vi "Begin.vi"(8 "error in":errorcluster) -> (0 "error out":errorcluster)   [LabVIEW 2020]
doc: "Called before other user functions, this VI is expected to open initial I/O refnums, load in file data, and do all program initialization. Notice that the <B>error out</B> terminal is simply used for data flow. Wiring it to other structures or subVIs ensures that this VI runs first."
uses:
  <vilib>/Rock Robotics/WPI/ThirdParty/Phoenix-LabVIEW/Motor Controller/Controls/CTRE_Phoenix_MotorControl_SupplyCurrentLimitConfiguration.ctl
  <vilib>/Rock Robotics/WPI/DriverStation/WPI_DriverStationRobotMode2.ctl
  <vilib>/Rock Robotics/WPI/Joystick/WPI_JoystickDeviceEnum.ctl
  <vilib>/Rock Robotics/WPI/ThirdParty/REV Robotics/REVLib/Typedef/Spark MAX Status Frames.ctl
  <vilib>/Rock Robotics/WPI/ThirdParty/Phoenix-LabVIEW/Motor Controller/Controls/CTRE_Phoenix_MotorControl_StatusFrameEnhanced.ctl
  <vilib>/Rock Robotics/SystemInterfaces/DIO/FPGA_DIOPWMChannel.ctl
  <vilib>/Rock Robotics/WPI/ThirdParty/REV Robotics/REVLib/Typedef/Spark MAX Control Type.ctl
  <vilib>/Rock Robotics/WPI/ThirdParty/Phoenix-LabVIEW/Motor Controller/Controls/CTRE_Phoenix_MotorControl_TalonFXInvertType.ctl
  <vilib>/Rock Robotics/WPI/ThirdParty/REV Robotics/REVLib/Typedef/Spark MAX Sensor Type.ctl
  <vilib>/Rock Robotics/WPI/ThirdParty/REV Robotics/REVLib/Typedef/Spark MAX Motor Type.ctl
  <vilib>/Rock Robotics/WPI/ThirdParty/REV Robotics/REVLib/Typedef/Spark MAX Idle Mode.ctl
  <vilib>/Rock Robotics/WPI/ThirdParty/Phoenix-LabVIEW/Motor Controller/Controls/CTRE_Phoenix_MotorControl_ControlFrameEnhanced.ctl
  <vilib>/Rock Robotics/WPI/ThirdParty/Phoenix-LabVIEW/Pigeon IMU/CTRE_PigeonIMU_StatusFrameRate.ctl
  <vilib>/Rock Robotics/WPI/ThirdParty/Phoenix-LabVIEW/Motor Controller/Controls/CTRE_Phoenix_MotorControl_NeutralMode.ctl
  Robot Global Data.vi
  <vilib>/Rock Robotics/WPI/ThirdParty/Phoenix-LabVIEW/Pigeon IMU/CTRE_PigeonIMU_Open_CAN.vi
panel:
  in  "Supply Current Limit Configuration":T1={"Enable?"=TRUE, "Current Limit"=30.0, "Threshold Current"=0.0, "Threshold Time"=0.0}
  in  "configPath":path=path "/home/lvuser/Config/config.ini"
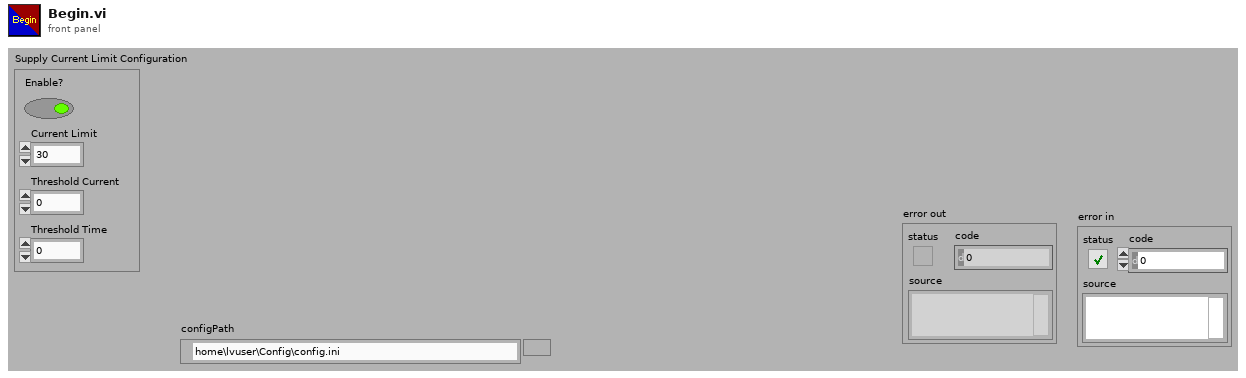
[diagram p1: front panel]
types:
  T1 = typedef "CTRE_Phoenix_MotorControl_SupplyCurrentLimitConfiguration.ctl" = cluster{"Enable?":bool, "Current Limit":dbl, "Threshold Current":dbl, "Threshold Time":dbl}
  T2 = typedef "WPI_DriverStationRobotMode2.ctl" = enum16{"Autonomous Disabled", "Autonomous Enabled", "Teleop Disabled", "Teleop Enabled", "Disconnected", "Finish", "Test Disabled", "Test Enabled", "Emergency Stopped"}
  T3 = typedef "CTRE_Phoenix_MotorControl_NeutralMode.ctl" = enum8{"EEPROMSetting", "Override to Coast", "Override to Brake"}
  T4 = typedef "Spark MAX Sensor Type.ctl" = enum16{"No Sensor", "Hall Sensor", "Encoder", "-Not Available-", "Analog", "Alternate Encoder"}
  T5 = typedef "CTRE_Phoenix_MotorControl_TalonFXInvertType.ctl" = enum16{"Counter-Clockwise", "Clockwise"}
  T6 = typedef "Spark MAX Status Frames.ctl" = enum16{"Status 0", "Status 1", "Status 2", "Status 3"}
  T7 = typedef "Spark MAX Idle Mode.ctl" = enum16{"Coast", "Brake"}
  T8 = typedef "Spark MAX Motor Type.ctl" = enum16{"Brushed", "Brushless"}
  T9 = cluster{"P Gain":dbl, "I Gain":dbl, "D Gain":dbl, "F Gain":dbl, "I Zone":dbl, "Min Output":dbl, "Max Output":dbl}
  T10 = typedef "Spark MAX Control Type.ctl" = enum16{"Percent VBus", "Voltage", "Velocity", "Position", "Smart Motion", "Current", "Smart Velocity"}
  T11 = typedef "FPGA_DIOPWMChannel.ctl" = enum8{"PWM 0", "PWM 1", "PWM 2", "PWM 3", "PWM 4", "PWM 5", "PWM 6", "PWM 7", "PWM 8", "PWM 9", "PWM MXP 0", "PWM MXP 1", "PWM MXP 2", "PWM MXP 3", "PWM MXP 4", "PWM MXP 5", "PWM MXP 6", "PWM MXP 7", "PWM MXP 8", "PWM MXP 9", "Invalid"}
  T12 = typedef "WPI_JoystickDeviceEnum.ctl" = enum16{"USB 0", "USB 1", "USB 2", "USB 3", "USB 4", "USB 5"}
  T13 = typedef "PiConfig.ctl" = cluster{"swerveModules":cluster{"leftFront":T14, "rightFront":T14, "leftRear":T14, "rightRear":T14}, "offsets":cluster{"leftFrontAngleOffset":dbl, "leftRearAngleOffset":dbl, "rightFrontAngleOffset":dbl, "rightRearAngleOffset":dbl}, "limits":cluster{"maxVelocity":dbl, "maxOverdriveVelocity":dbl, "maxAcceleration":dbl, "maxPickupVelocity":dbl, "maxClimbArmVelocity":dbl}, "speeds":cluster{"intakeSuckSpeed":dbl, "intakeSpitSpeed":dbl, "indexerSuckSpeed":dbl, "indexerSpitSpeed":dbl, "indexerShootSpeed":dbl, "indexerBumpBackSpeed":dbl, "shooterSpinupSpeed":dbl, "kickupSpinupSpeed":dbl, "shooterLowShootSpeed":dbl, "shooterHighShootSpeed":dbl, "shooterPadSpeed":dbl, "shooterWallSpeed":dbl}, "positions":cluster{"intakeStarting":dbl, "intakeStow":dbl, "intakeSuck":dbl, "armPounce":dbl, "armStow":dbl, "armUp":dbl, "winchPounce":dbl, "winchOut":dbl, "winchStow":dbl, "intakeSpit":dbl, "winchBarEngage":dbl, "winchBottomClimb":dbl, "hoodHighShoot":dbl, "armClearHooks":dbl, "winchClearHooks":dbl, "armLiftNextBar":dbl, "winchEngageHooksNextBar":dbl, "winchEngagePassive":dbl, "winchTraversalClimb":dbl, "hoodPadShoot":dbl, "turretPadShoot":dbl, "hoodWallShoot":dbl, "turretWallShoot":dbl, "winchRobotOffBar":dbl, "winchSettleClimb":dbl}, "inversions":cluster{"rightShooter":bool, "leftShooter":bool}}
  T14 = typedef "Swerve Module Parameters.ctl" = cluster{"driveCANID":dbl, "angleCANID":i32, "canCoderCANID":dbl, "moduleName":string, "driveMotorNeutralMode":T3, "driveCurrentLimitConfig":T1, "driveFeedbackDevice":T15, "driveInitialSensorPosition":dbl, "driveEnableVoltageComp":bool, "driveVoltageComp":dbl, "driveRampRate":dbl, "angleCurrentLimit":dbl, "angleSensorType":T4, "angleMotorType":T8, "angleConversionFactor":dbl, "anglePIDRamp":dbl, "angleVoltageComp":dbl, "angleIdleMode":T7, "cancoderConfig":T16, "angleInitialSensorPosition":dbl}
  T15 = typedef "CTRE_Phoenix_MotorControl_FeedbackDevice_TalonFX.ctl" = i8
  T16 = typedef "CTRE_Phoenix_CANcoder_Configurables.ctl" = cluster{"Sensor Initialization Strategy":T17, "Absolute Sensor Range":T18, "Velocity Measurement Period":T19, "Velocity Measurement Window":i32, "Magnet Offset (Degrees)":dbl, "Sensor Direction":bool, "Sensor Coefficient":dbl, "Unit String":string, "Sensor Time Base":T20}
  T17 = typedef "CTRE_Phoenix_CANcoder_SensorInitializationStrategy.ctl" = enum16{"Boot To Zero", "Boot To Absolute Position"}
  T18 = typedef "CTRE_Phoenix_CANcoder_AbsoluteSensorRange.ctl" = enum16{"Unsigned [0 to 360)", "Signed [-180 to +180)"}
  T19 = typedef "CTRE_Phoenix_MotorControl_VelocityMeasurementPeriod.ctl" = u16
  T20 = typedef "CTRE_Phoenix_CANcoder_SensorTimeBase.ctl" = enum16{"Per100Ms_Legacy", "PerSecond", "PerMinute"}
  T21 = typedef "CTRE_Phoenix_MotorControl_ControlFrameEnhanced.ctl" = u32
  T22 = typedef "CTRE_Phoenix_MotorControl_StatusFrameEnhanced.ctl" = u16
  T23 = typedef "CTRE_PigeonIMU_StatusFrameRate.ctl" = u32
  T24 = typedef "WPI_JoystickDevRef.ctl" = cluster{"Device":T12}
  T25 = typedef "WPI_ServoDeviceRef.ctl" = cluster{"DeviceStatus":errorcluster, "PWM Channel":T11, "DeadBand":T26}
  T26 = typedef "WPI_PWMDeadband.ctl" = cluster{"Name":string, "maxPositivePwm":i32, "minPositivePwm":i32, "centerPwm":i32, "maxNegativePwm":i32, "minNegativePwm":i32, "angularRange":u16}
  T27 = typedef "CTRE_PigeonIMU_DeviceRef.ctl" = cluster{"DeviceStatus":errorcluster, "Device Number":u8, "Type":T28, "Device ID":u32, "Handle":u64, "UsageFrame":u32, "Library Path":path}
  T28 = typedef "CTRE_PigeonIMU_ConnectionType.ctl" = u32
  T29 = typedef "WPI_MotorControlDeviceRef.ctl" = cluster{"DeviceStatus":errorcluster, "Type":T30, "PWM":cluster{"PWM Channel":T11, "DeadBand":T26}, "CAN":cluster{"Device Number":u8, "SetOutput VI Ref":variant, "GetOutput VI Ref":variant, "Enable VI Ref":variant, "Disable VI Ref":variant, "Data":variant}, "Invert":bool, "DIO PWM":cluster{"PWM \"Enable\" Channel":T11, "DIOChannel":T31, "PWM Rate":dbl}}
  T30 = typedef "WPI_MotorControlType.ctl" = enum16{"PWM", "CAN", "DIO PWM"}
  T31 = typedef "FPGA_DIOChannel.ctl" = enum8{"DIO 0", "DIO 1", "DIO 2", "DIO 3", "DIO 4", "DIO 5", "DIO 6", "DIO 7", "DIO 8", "DIO 9", "DIO MXP 0", "DIO MXP 1", "DIO MXP 2", "DIO MXP 3", "DIO MXP 4", "DIO MXP 5", "DIO MXP 6", "DIO MXP 7", "DIO MXP 8", "DIO MXP 9", "DIO MXP 10", "DIO MXP 11", "DIO MXP 12", "DIO MXP 13", "DIO MXP 14", "DIO MXP 15", "SPI Port CS1", "SPI Port CS2", "SPI Port CS3", "SPI Port MISO", "SPI Port MOSI", "Invalid"}
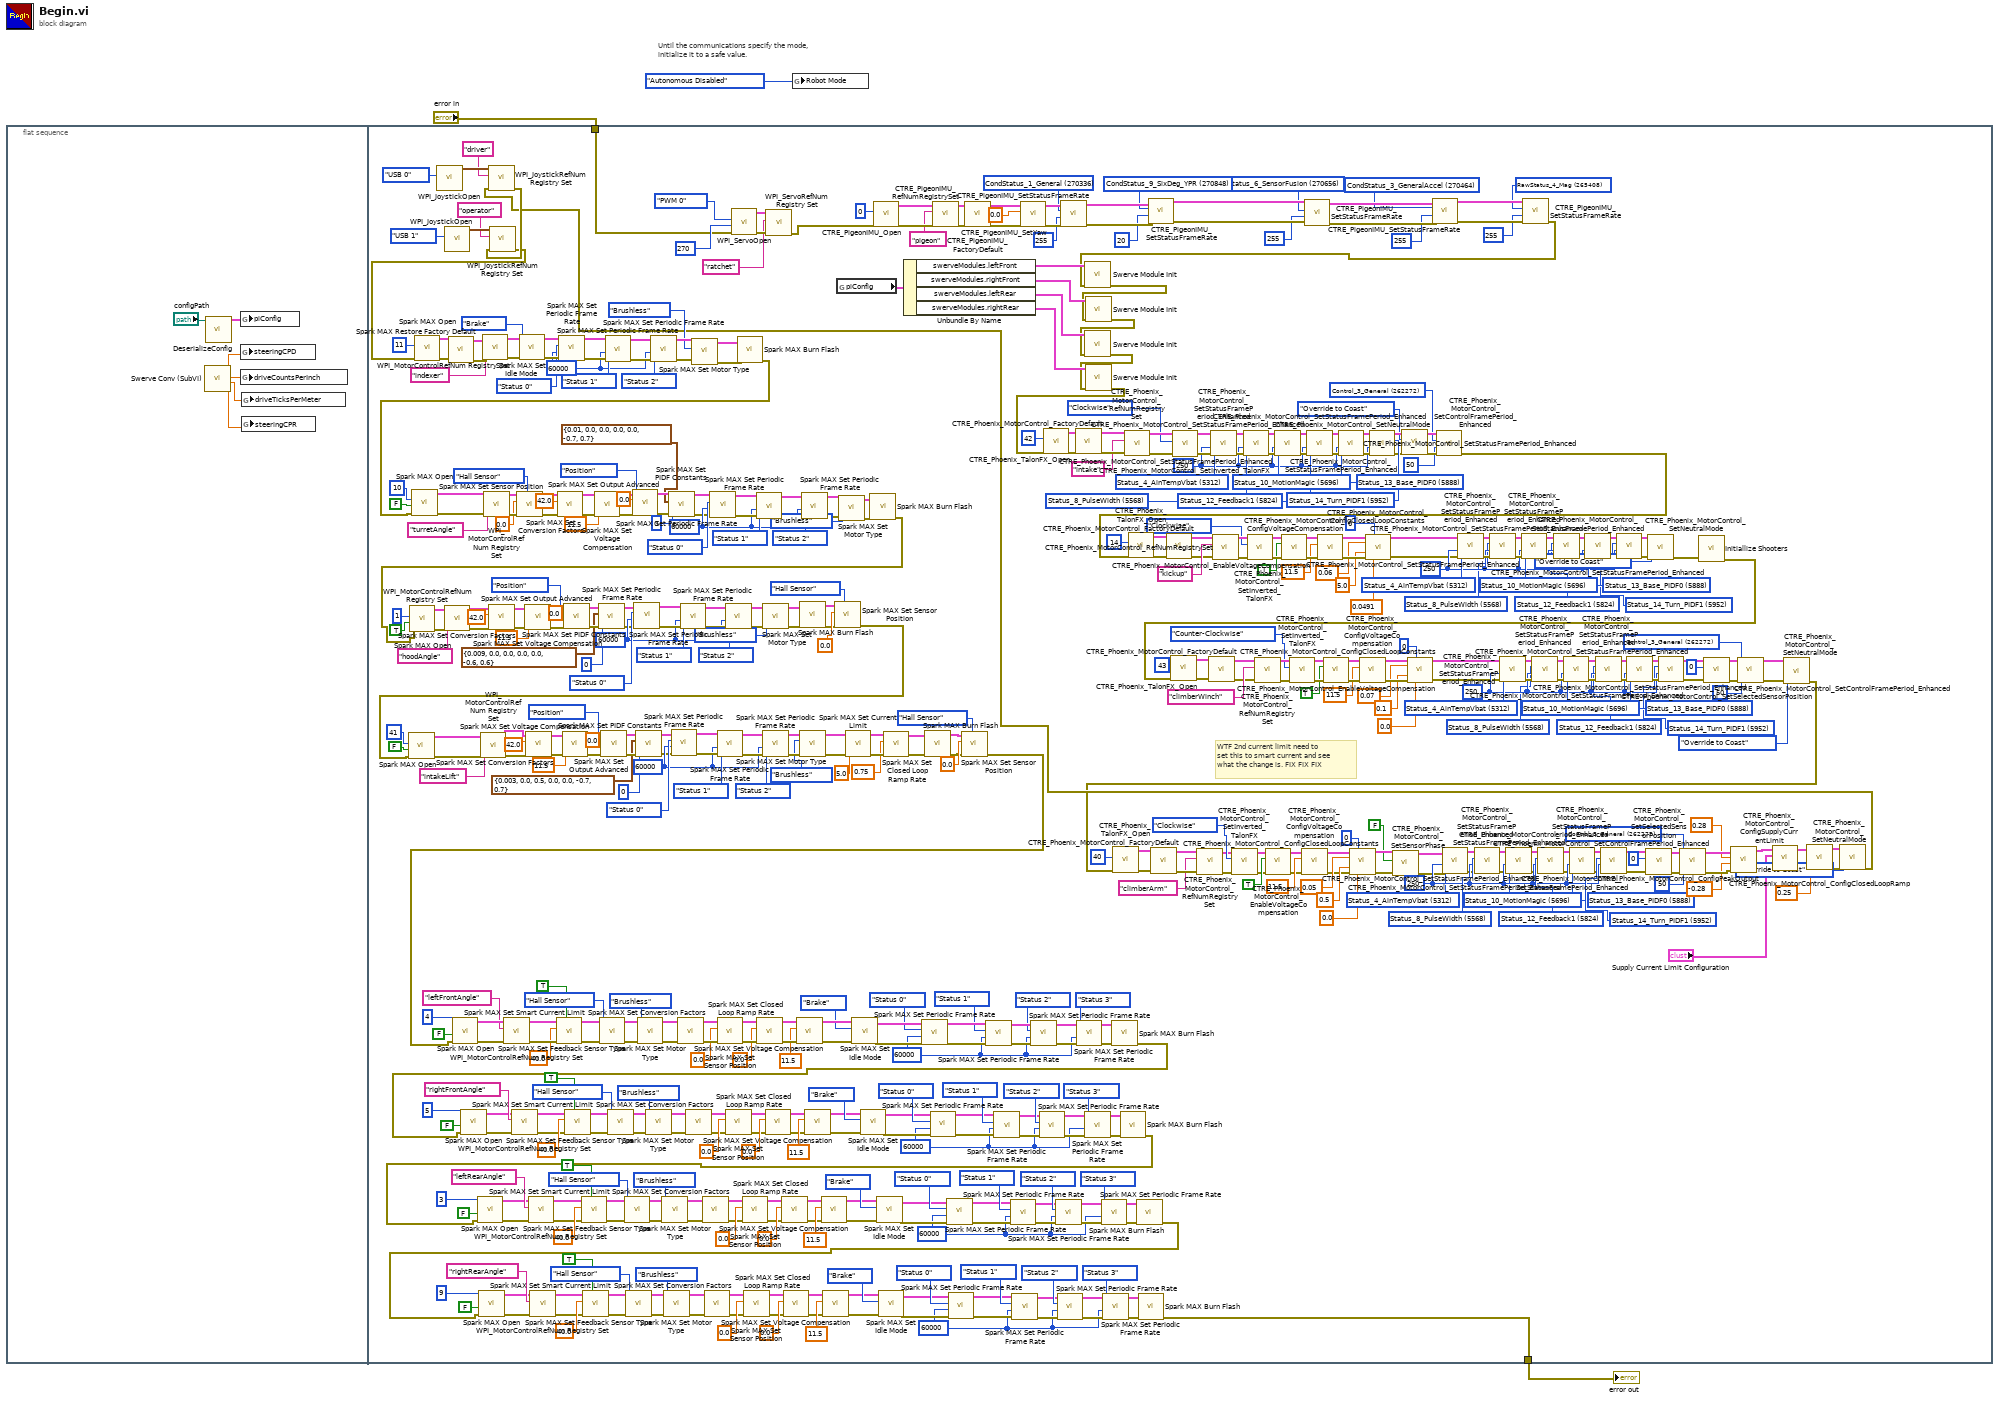
[diagram p0: block diagram]
diagram:
  # "Until the communications specify the mode,\ninitialize it to a safe value."
  n1 = flat-sequence {
    tunnel: "error in" -> [w97]
    tunnel: [w91] -> w1
    frame #0 {
      n2 = call "Swerve Conv (SubVI).vi"() -> ("steeringModuleCPR"=w8:dbl, "driveCountsPerMeter"=w4:dbl, "driveCountsPerInch"=w6:dbl, "steeringModuleCPD"=w7:dbl)  [unwired: 8 in]
      n3 = call "DeserializeConfig.vi"("configPath"="configPath") -> ("config"=w9:T13)  [unwired: 10 in]
      n4 = global write "Robot Global Data.vi" "piConfig"(w9) -> ()
      n5 = global write "Robot Global Data.vi" "steeringCPD"(w7) -> ()
      n6 = global write "Robot Global Data.vi" "driveCountsPerInch"(w6) -> ()
      n7 = global write "Robot Global Data.vi" "driveTicksPerMeter"(w4) -> ()
      n8 = global write "Robot Global Data.vi" "steeringCPR"(w8) -> ()
    }
    frame #1 {
      w89 = T21 262272 items=["Control_3_General"=262272, "Control_4_Advanced"=262336, "Control_5_FeedbackOutputOverride"=262400, "Control_6_MotProfAddTrajPoint"=262464] ("Control Frame")
      w77 = 250 ("periodMs")
      w80 = T22 5952 items=["Status_1_General"=5120, "Status_2_Feedback0"=5184, "Status_3_Quadrature"=5248, "Status_4_AinTempVbat"=5312, "Status_6_Misc"=5440, "Status_7_CommStatus"=5504, "Status_8_PulseWidth"=5568, "Status_9_MotProfBuffer"=5632, "Status_10_MotionMagic"=5696, "Status_11_UartGadgeteer"=5760, "Status_12_Feedback1"=5824, "Status_13_Base_PIDF0"=5888, "Status_14_Turn_PIDF1"=5952, "Status_15_FirmwareApiStatus"=6016, "Status_Brushless_Current"=4672] ("Status Frame")
      w76 = T22 5888 items=["Status_1_General"=5120, "Status_2_Feedback0"=5184, "Status_3_Quadrature"=5248, "Status_4_AinTempVbat"=5312, "Status_6_Misc"=5440, "Status_7_CommStatus"=5504, "Status_8_PulseWidth"=5568, "Status_9_MotProfBuffer"=5632, "Status_10_MotionMagic"=5696, "Status_11_UartGadgeteer"=5760, "Status_12_Feedback1"=5824, "Status_13_Base_PIDF0"=5888, "Status_14_Turn_PIDF1"=5952, "Status_15_FirmwareApiStatus"=6016, "Status_Brushless_Current"=4672] ("Status Frame")
      w79 = T22 5824 items=["Status_1_General"=5120, "Status_2_Feedback0"=5184, "Status_3_Quadrature"=5248, "Status_4_AinTempVbat"=5312, "Status_6_Misc"=5440, "Status_7_CommStatus"=5504, "Status_8_PulseWidth"=5568, "Status_9_MotProfBuffer"=5632, "Status_10_MotionMagic"=5696, "Status_11_UartGadgeteer"=5760, "Status_12_Feedback1"=5824, "Status_13_Base_PIDF0"=5888, "Status_14_Turn_PIDF1"=5952, "Status_15_FirmwareApiStatus"=6016, "Status_Brushless_Current"=4672] ("Status Frame")
      w75 = T22 5696 items=["Status_1_General"=5120, "Status_2_Feedback0"=5184, "Status_3_Quadrature"=5248, "Status_4_AinTempVbat"=5312, "Status_6_Misc"=5440, "Status_7_CommStatus"=5504, "Status_8_PulseWidth"=5568, "Status_9_MotProfBuffer"=5632, "Status_10_MotionMagic"=5696, "Status_11_UartGadgeteer"=5760, "Status_12_Feedback1"=5824, "Status_13_Base_PIDF0"=5888, "Status_14_Turn_PIDF1"=5952, "Status_15_FirmwareApiStatus"=6016, "Status_Brushless_Current"=4672] ("Status Frame")
      w78 = T22 5568 items=["Status_1_General"=5120, "Status_2_Feedback0"=5184, "Status_3_Quadrature"=5248, "Status_4_AinTempVbat"=5312, "Status_6_Misc"=5440, "Status_7_CommStatus"=5504, "Status_8_PulseWidth"=5568, "Status_9_MotProfBuffer"=5632, "Status_10_MotionMagic"=5696, "Status_11_UartGadgeteer"=5760, "Status_12_Feedback1"=5824, "Status_13_Base_PIDF0"=5888, "Status_14_Turn_PIDF1"=5952, "Status_15_FirmwareApiStatus"=6016, "Status_Brushless_Current"=4672] ("Status Frame")
      w74 = T22 5312 items=["Status_1_General"=5120, "Status_2_Feedback0"=5184, "Status_3_Quadrature"=5248, "Status_4_AinTempVbat"=5312, "Status_6_Misc"=5440, "Status_7_CommStatus"=5504, "Status_8_PulseWidth"=5568, "Status_9_MotProfBuffer"=5632, "Status_10_MotionMagic"=5696, "Status_11_UartGadgeteer"=5760, "Status_12_Feedback1"=5824, "Status_13_Base_PIDF0"=5888, "Status_14_Turn_PIDF1"=5952, "Status_15_FirmwareApiStatus"=6016, "Status_Brushless_Current"=4672] ("Status Frame")
      w102 = T23 265408 items=["CondStatus_1_General"=270336, "CondStatus_9_SixDeg_YPR"=270848, "CondStatus_6_SensorFusion"=270656, "CondStatus_11_GyroAccum"=270976, "CondStatus_2_GeneralCompass"=270400, "CondStatus_3_GeneralAccel"=270464, "CondStatus_10_SixDeg_Quat"=270912, "RawStatus_4_Mag"=265408, "BiasedStatus_2_Gyro"=269376, "BiasedStatus_4_Mag"=269504, "BiasedStatus_6_Accel"=269632] ("StatusFrame")
      w103 = T23 270464 items=["CondStatus_1_General"=270336, "CondStatus_9_SixDeg_YPR"=270848, "CondStatus_6_SensorFusion"=270656, "CondStatus_11_GyroAccum"=270976, "CondStatus_2_GeneralCompass"=270400, "CondStatus_3_GeneralAccel"=270464, "CondStatus_10_SixDeg_Quat"=270912, "RawStatus_4_Mag"=265408, "BiasedStatus_2_Gyro"=269376, "BiasedStatus_4_Mag"=269504, "BiasedStatus_6_Accel"=269632] ("StatusFrame")
      w104 = T23 270656 items=["CondStatus_1_General"=270336, "CondStatus_9_SixDeg_YPR"=270848, "CondStatus_6_SensorFusion"=270656, "CondStatus_11_GyroAccum"=270976, "CondStatus_2_GeneralCompass"=270400, "CondStatus_3_GeneralAccel"=270464, "CondStatus_10_SixDeg_Quat"=270912, "RawStatus_4_Mag"=265408, "BiasedStatus_2_Gyro"=269376, "BiasedStatus_4_Mag"=269504, "BiasedStatus_6_Accel"=269632] ("StatusFrame")
      w105 = T23 270848 items=["CondStatus_1_General"=270336, "CondStatus_9_SixDeg_YPR"=270848, "CondStatus_6_SensorFusion"=270656, "CondStatus_11_GyroAccum"=270976, "CondStatus_2_GeneralCompass"=270400, "CondStatus_3_GeneralAccel"=270464, "CondStatus_10_SixDeg_Quat"=270912, "RawStatus_4_Mag"=265408, "BiasedStatus_2_Gyro"=269376, "BiasedStatus_4_Mag"=269504, "BiasedStatus_6_Accel"=269632] ("StatusFrame")
      w115 = T23 270336 items=["CondStatus_1_General"=270336, "CondStatus_9_SixDeg_YPR"=270848, "CondStatus_6_SensorFusion"=270656, "CondStatus_11_GyroAccum"=270976, "CondStatus_2_GeneralCompass"=270400, "CondStatus_3_GeneralAccel"=270464, "CondStatus_10_SixDeg_Quat"=270912, "RawStatus_4_Mag"=265408, "BiasedStatus_2_Gyro"=269376, "BiasedStatus_4_Mag"=269504, "BiasedStatus_6_Accel"=269632] ("StatusFrame")
      w119 = T21 262272 items=["Control_3_General"=262272, "Control_4_Advanced"=262336, "Control_5_FeedbackOutputOverride"=262400, "Control_6_MotProfAddTrajPoint"=262464] ("Control Frame")
      w123 = T21 262272 items=["Control_3_General"=262272, "Control_4_Advanced"=262336, "Control_5_FeedbackOutputOverride"=262400, "Control_6_MotProfAddTrajPoint"=262464] ("Control Frame")
      w131 = u16 60000 ("Frame rate (ms)")
      w132 = u16 60000 ("Frame rate (ms)")
      w133 = u16 60000 ("Frame rate (ms)")
      w134 = u16 60000 ("Frame rate (ms)")
      w332 = 250 ("periodMs")
      w329 = T22 5952 items=["Status_1_General"=5120, "Status_2_Feedback0"=5184, "Status_3_Quadrature"=5248, "Status_4_AinTempVbat"=5312, "Status_6_Misc"=5440, "Status_7_CommStatus"=5504, "Status_8_PulseWidth"=5568, "Status_9_MotProfBuffer"=5632, "Status_10_MotionMagic"=5696, "Status_11_UartGadgeteer"=5760, "Status_12_Feedback1"=5824, "Status_13_Base_PIDF0"=5888, "Status_14_Turn_PIDF1"=5952, "Status_15_FirmwareApiStatus"=6016, "Status_Brushless_Current"=4672] ("Status Frame")
      w333 = T22 5888 items=["Status_1_General"=5120, "Status_2_Feedback0"=5184, "Status_3_Quadrature"=5248, "Status_4_AinTempVbat"=5312, "Status_6_Misc"=5440, "Status_7_CommStatus"=5504, "Status_8_PulseWidth"=5568, "Status_9_MotProfBuffer"=5632, "Status_10_MotionMagic"=5696, "Status_11_UartGadgeteer"=5760, "Status_12_Feedback1"=5824, "Status_13_Base_PIDF0"=5888, "Status_14_Turn_PIDF1"=5952, "Status_15_FirmwareApiStatus"=6016, "Status_Brushless_Current"=4672] ("Status Frame")
      w330 = T22 5824 items=["Status_1_General"=5120, "Status_2_Feedback0"=5184, "Status_3_Quadrature"=5248, "Status_4_AinTempVbat"=5312, "Status_6_Misc"=5440, "Status_7_CommStatus"=5504, "Status_8_PulseWidth"=5568, "Status_9_MotProfBuffer"=5632, "Status_10_MotionMagic"=5696, "Status_11_UartGadgeteer"=5760, "Status_12_Feedback1"=5824, "Status_13_Base_PIDF0"=5888, "Status_14_Turn_PIDF1"=5952, "Status_15_FirmwareApiStatus"=6016, "Status_Brushless_Current"=4672] ("Status Frame")
      w334 = T22 5696 items=["Status_1_General"=5120, "Status_2_Feedback0"=5184, "Status_3_Quadrature"=5248, "Status_4_AinTempVbat"=5312, "Status_6_Misc"=5440, "Status_7_CommStatus"=5504, "Status_8_PulseWidth"=5568, "Status_9_MotProfBuffer"=5632, "Status_10_MotionMagic"=5696, "Status_11_UartGadgeteer"=5760, "Status_12_Feedback1"=5824, "Status_13_Base_PIDF0"=5888, "Status_14_Turn_PIDF1"=5952, "Status_15_FirmwareApiStatus"=6016, "Status_Brushless_Current"=4672] ("Status Frame")
      w331 = T22 5568 items=["Status_1_General"=5120, "Status_2_Feedback0"=5184, "Status_3_Quadrature"=5248, "Status_4_AinTempVbat"=5312, "Status_6_Misc"=5440, "Status_7_CommStatus"=5504, "Status_8_PulseWidth"=5568, "Status_9_MotProfBuffer"=5632, "Status_10_MotionMagic"=5696, "Status_11_UartGadgeteer"=5760, "Status_12_Feedback1"=5824, "Status_13_Base_PIDF0"=5888, "Status_14_Turn_PIDF1"=5952, "Status_15_FirmwareApiStatus"=6016, "Status_Brushless_Current"=4672] ("Status Frame")
      w335 = T22 5312 items=["Status_1_General"=5120, "Status_2_Feedback0"=5184, "Status_3_Quadrature"=5248, "Status_4_AinTempVbat"=5312, "Status_6_Misc"=5440, "Status_7_CommStatus"=5504, "Status_8_PulseWidth"=5568, "Status_9_MotProfBuffer"=5632, "Status_10_MotionMagic"=5696, "Status_11_UartGadgeteer"=5760, "Status_12_Feedback1"=5824, "Status_13_Base_PIDF0"=5888, "Status_14_Turn_PIDF1"=5952, "Status_15_FirmwareApiStatus"=6016, "Status_Brushless_Current"=4672] ("Status Frame")
      w370 = u16 60000 ("Frame rate (ms)")
      w421 = 250 ("periodMs")
      w418 = T22 5952 items=["Status_1_General"=5120, "Status_2_Feedback0"=5184, "Status_3_Quadrature"=5248, "Status_4_AinTempVbat"=5312, "Status_6_Misc"=5440, "Status_7_CommStatus"=5504, "Status_8_PulseWidth"=5568, "Status_9_MotProfBuffer"=5632, "Status_10_MotionMagic"=5696, "Status_11_UartGadgeteer"=5760, "Status_12_Feedback1"=5824, "Status_13_Base_PIDF0"=5888, "Status_14_Turn_PIDF1"=5952, "Status_15_FirmwareApiStatus"=6016, "Status_Brushless_Current"=4672] ("Status Frame")
      w422 = T22 5888 items=["Status_1_General"=5120, "Status_2_Feedback0"=5184, "Status_3_Quadrature"=5248, "Status_4_AinTempVbat"=5312, "Status_6_Misc"=5440, "Status_7_CommStatus"=5504, "Status_8_PulseWidth"=5568, "Status_9_MotProfBuffer"=5632, "Status_10_MotionMagic"=5696, "Status_11_UartGadgeteer"=5760, "Status_12_Feedback1"=5824, "Status_13_Base_PIDF0"=5888, "Status_14_Turn_PIDF1"=5952, "Status_15_FirmwareApiStatus"=6016, "Status_Brushless_Current"=4672] ("Status Frame")
      w419 = T22 5824 items=["Status_1_General"=5120, "Status_2_Feedback0"=5184, "Status_3_Quadrature"=5248, "Status_4_AinTempVbat"=5312, "Status_6_Misc"=5440, "Status_7_CommStatus"=5504, "Status_8_PulseWidth"=5568, "Status_9_MotProfBuffer"=5632, "Status_10_MotionMagic"=5696, "Status_11_UartGadgeteer"=5760, "Status_12_Feedback1"=5824, "Status_13_Base_PIDF0"=5888, "Status_14_Turn_PIDF1"=5952, "Status_15_FirmwareApiStatus"=6016, "Status_Brushless_Current"=4672] ("Status Frame")
      w423 = T22 5696 items=["Status_1_General"=5120, "Status_2_Feedback0"=5184, "Status_3_Quadrature"=5248, "Status_4_AinTempVbat"=5312, "Status_6_Misc"=5440, "Status_7_CommStatus"=5504, "Status_8_PulseWidth"=5568, "Status_9_MotProfBuffer"=5632, "Status_10_MotionMagic"=5696, "Status_11_UartGadgeteer"=5760, "Status_12_Feedback1"=5824, "Status_13_Base_PIDF0"=5888, "Status_14_Turn_PIDF1"=5952, "Status_15_FirmwareApiStatus"=6016, "Status_Brushless_Current"=4672] ("Status Frame")
      w420 = T22 5568 items=["Status_1_General"=5120, "Status_2_Feedback0"=5184, "Status_3_Quadrature"=5248, "Status_4_AinTempVbat"=5312, "Status_6_Misc"=5440, "Status_7_CommStatus"=5504, "Status_8_PulseWidth"=5568, "Status_9_MotProfBuffer"=5632, "Status_10_MotionMagic"=5696, "Status_11_UartGadgeteer"=5760, "Status_12_Feedback1"=5824, "Status_13_Base_PIDF0"=5888, "Status_14_Turn_PIDF1"=5952, "Status_15_FirmwareApiStatus"=6016, "Status_Brushless_Current"=4672] ("Status Frame")
      w424 = T22 5312 items=["Status_1_General"=5120, "Status_2_Feedback0"=5184, "Status_3_Quadrature"=5248, "Status_4_AinTempVbat"=5312, "Status_6_Misc"=5440, "Status_7_CommStatus"=5504, "Status_8_PulseWidth"=5568, "Status_9_MotProfBuffer"=5632, "Status_10_MotionMagic"=5696, "Status_11_UartGadgeteer"=5760, "Status_12_Feedback1"=5824, "Status_13_Base_PIDF0"=5888, "Status_14_Turn_PIDF1"=5952, "Status_15_FirmwareApiStatus"=6016, "Status_Brushless_Current"=4672] ("Status Frame")
      w435 = 250 ("periodMs")
      w436 = T22 5952 items=["Status_1_General"=5120, "Status_2_Feedback0"=5184, "Status_3_Quadrature"=5248, "Status_4_AinTempVbat"=5312, "Status_6_Misc"=5440, "Status_7_CommStatus"=5504, "Status_8_PulseWidth"=5568, "Status_9_MotProfBuffer"=5632, "Status_10_MotionMagic"=5696, "Status_11_UartGadgeteer"=5760, "Status_12_Feedback1"=5824, "Status_13_Base_PIDF0"=5888, "Status_14_Turn_PIDF1"=5952, "Status_15_FirmwareApiStatus"=6016, "Status_Brushless_Current"=4672] ("Status Frame")
      w437 = T22 5888 items=["Status_1_General"=5120, "Status_2_Feedback0"=5184, "Status_3_Quadrature"=5248, "Status_4_AinTempVbat"=5312, "Status_6_Misc"=5440, "Status_7_CommStatus"=5504, "Status_8_PulseWidth"=5568, "Status_9_MotProfBuffer"=5632, "Status_10_MotionMagic"=5696, "Status_11_UartGadgeteer"=5760, "Status_12_Feedback1"=5824, "Status_13_Base_PIDF0"=5888, "Status_14_Turn_PIDF1"=5952, "Status_15_FirmwareApiStatus"=6016, "Status_Brushless_Current"=4672] ("Status Frame")
      w438 = T22 5824 items=["Status_1_General"=5120, "Status_2_Feedback0"=5184, "Status_3_Quadrature"=5248, "Status_4_AinTempVbat"=5312, "Status_6_Misc"=5440, "Status_7_CommStatus"=5504, "Status_8_PulseWidth"=5568, "Status_9_MotProfBuffer"=5632, "Status_10_MotionMagic"=5696, "Status_11_UartGadgeteer"=5760, "Status_12_Feedback1"=5824, "Status_13_Base_PIDF0"=5888, "Status_14_Turn_PIDF1"=5952, "Status_15_FirmwareApiStatus"=6016, "Status_Brushless_Current"=4672] ("Status Frame")
      w439 = T22 5696 items=["Status_1_General"=5120, "Status_2_Feedback0"=5184, "Status_3_Quadrature"=5248, "Status_4_AinTempVbat"=5312, "Status_6_Misc"=5440, "Status_7_CommStatus"=5504, "Status_8_PulseWidth"=5568, "Status_9_MotProfBuffer"=5632, "Status_10_MotionMagic"=5696, "Status_11_UartGadgeteer"=5760, "Status_12_Feedback1"=5824, "Status_13_Base_PIDF0"=5888, "Status_14_Turn_PIDF1"=5952, "Status_15_FirmwareApiStatus"=6016, "Status_Brushless_Current"=4672] ("Status Frame")
      w440 = T22 5568 items=["Status_1_General"=5120, "Status_2_Feedback0"=5184, "Status_3_Quadrature"=5248, "Status_4_AinTempVbat"=5312, "Status_6_Misc"=5440, "Status_7_CommStatus"=5504, "Status_8_PulseWidth"=5568, "Status_9_MotProfBuffer"=5632, "Status_10_MotionMagic"=5696, "Status_11_UartGadgeteer"=5760, "Status_12_Feedback1"=5824, "Status_13_Base_PIDF0"=5888, "Status_14_Turn_PIDF1"=5952, "Status_15_FirmwareApiStatus"=6016, "Status_Brushless_Current"=4672] ("Status Frame")
      w441 = T22 5312 items=["Status_1_General"=5120, "Status_2_Feedback0"=5184, "Status_3_Quadrature"=5248, "Status_4_AinTempVbat"=5312, "Status_6_Misc"=5440, "Status_7_CommStatus"=5504, "Status_8_PulseWidth"=5568, "Status_9_MotProfBuffer"=5632, "Status_10_MotionMagic"=5696, "Status_11_UartGadgeteer"=5760, "Status_12_Feedback1"=5824, "Status_13_Base_PIDF0"=5888, "Status_14_Turn_PIDF1"=5952, "Status_15_FirmwareApiStatus"=6016, "Status_Brushless_Current"=4672] ("Status Frame")
      w458 = u16 60000 ("Frame rate (ms)")
      w466 = u16 60000 ("Frame rate (ms)")
      w474 = u16 60000 ("Frame rate (ms)")
      # "WTF 2nd current limit need to\nset this to smart current and see\nwhat the change is. FIX FIX FIX"
      n9 = call <vilib>:"WPI_JoystickOpen.vi"("JoystickDevice"=WPI_JoystickDeviceEnum."USB 0") -> ("JoystickDevRef"=w578:T24)  [unwired: 10 in]
      n10 = call <vilib>:"WPI_JoystickOpen.vi"("JoystickDevice"=WPI_JoystickDeviceEnum."USB 1") -> ("JoystickDevRef"=w579:T24)  [unwired: 10 in]
      n11 = call <vilib>:"WPI_ServoOpen.vi"("error in (no error)"=w97, "Angular Range"=u16 270, "PWM Channel"=FPGA_DIOPWMChannel."PWM 0") -> ("error out"=w397:errorcluster, "ServoDeviceRef"=w396:T25)  [unwired: 7 in]
      n12 = call <vilib>:"WPI_ServoRefNum Registry Set.vi"("error in (no error)"=w397, "refnum name"="ratchet", "ServoDeviceRef"=w396) -> ("error out"=w96:errorcluster)  [unwired: 7 in, 1 out]
      n13 = global read "Robot Global Data.vi" "piConfig"() -> (w573:T13)
      n14 = call-poly <vilib>:"CTRE_PigeonIMU_Open.vi"("error in"=w96, "Device Number"=u8 0) -> ("error out"=w582:errorcluster, "PigeonIMUDevRef"=w583:T27)  [unwired: 8 in]
      n15 = Unbundle By Name(w573) -> ("swerveModules.leftFront"=w572:T14, "swerveModules.rightFront"=w571:T14, "swerveModules.leftRear"=w569:T14, "swerveModules.rightRear"=w570:T14)
      n16 = call <vilib>:"CTRE_PigeonIMU_RefNumRegistrySet.vi"("error in (no error)"=w582, "refnum name"="pigeon", "PigeonIMUDevRef"=w583) -> ("error out"=w584:errorcluster, "PigeonIMUDevRef"=w585:T27)  [unwired: 7 in]
      n17 = call <vilib>:"CTRE_PigeonIMU_FactoryDefault.vi"("error in"=w584, "PigeonIMUDevRef"=w585) -> ("error out"=w586:errorcluster, "PigeonIMUDevRef"=w587:T27)  [unwired: 8 in]
      n18 = call <vilib>:"CTRE_PigeonIMU_SetYaw.vi"("error in (no error)"=w586, "Value"=0.0, "PigeonIMUDevRef"=w587) -> ("error out"=w117:errorcluster, "PigeonIMUDevRef"=w116:T27)  [unwired: 7 in]
      n19 = call <vilib>:"CTRE_PigeonIMU_SetStatusFrameRate.vi"("error in (no error)"=w117, "Period (ms)"=i16 255, "StatusFrame"=w115, "PigeonIMUDevRef"=w116) -> ("error out"=w111:errorcluster, "PigeonIMUDevRef"=w112:T27)  [unwired: 6 in]
      n20 = call <vilib>:"CTRE_PigeonIMU_SetStatusFrameRate.vi"("error in (no error)"=w111, "Period (ms)"=i16 20, "StatusFrame"=w105, "PigeonIMUDevRef"=w112) -> ("error out"=w109:errorcluster, "PigeonIMUDevRef"=w110:T27)  [unwired: 6 in]
      n21 = call <vilib>:"CTRE_PigeonIMU_SetStatusFrameRate.vi"("error in (no error)"=w109, "Period (ms)"=i16 255, "StatusFrame"=w104, "PigeonIMUDevRef"=w110) -> ("error out"=w114:errorcluster, "PigeonIMUDevRef"=w113:T27)  [unwired: 6 in]
      n22 = call <vilib>:"CTRE_PigeonIMU_SetStatusFrameRate.vi"("error in (no error)"=w114, "Period (ms)"=i16 255, "StatusFrame"=w103, "PigeonIMUDevRef"=w113) -> ("error out"=w107:errorcluster, "PigeonIMUDevRef"=w108:T27)  [unwired: 6 in]
      n23 = call <vilib>:"CTRE_PigeonIMU_SetStatusFrameRate.vi"("error in (no error)"=w107, "Period (ms)"=i16 255, "StatusFrame"=w102, "PigeonIMUDevRef"=w108) -> ("error out"=w95:errorcluster)  [unwired: 6 in, 1 out]
      n24 = call "Swerve Module Init.vi"("error in"=w95, "swerveModuleParameters"=w572) -> ("error out"=w106:errorcluster)  [unwired: 9 in]
      n25 = call "Swerve Module Init.vi"("error in"=w106, "swerveModuleParameters"=w571) -> ("error out"=w567:errorcluster)  [unwired: 9 in]
      n26 = call "Swerve Module Init.vi"("error in"=w567, "swerveModuleParameters"=w569) -> ("error out"=w566:errorcluster)  [unwired: 9 in]
      n27 = call "Swerve Module Init.vi"("error in"=w566, "swerveModuleParameters"=w570) -> ("error out"=w543:errorcluster)  [unwired: 9 in]
      n28 = call <vilib>:"CTRE_Phoenix_TalonFX_Open.vi"("error in"=w543, "Device Number"=u8 42) -> ("error out"=w564:errorcluster, "PhoenixMotorControlDevRef"=w563:T29)  [unwired: 8 in]
      n29 = call <vilib>:"CTRE_Phoenix_MotorControl_FactoryDefault.vi"("error in"=w564, "PhoenixMotorControlDevRef"=w563) -> ("error out"=w562:errorcluster, "PhoenixMotorControlDevRef"=w561:T29)  [unwired: 8 in]
      n30 = call <vilib>:"CTRE_Phoenix_MotorControl_RefNumRegistrySet.vi"("error in (no error)"=w562, "refnum name"="intake", "PhoenixMotorControlDevRef"=w561) -> ("error out"=w542:errorcluster, "PhoenixMotorControlDevRef"=w541:T29)  [unwired: 7 in]
      n31 = call <vilib>:"CTRE_Phoenix_MotorControl_SetInverted_TalonFX.vi"("error in (no error)"=w542, "Invert Type"=CTRE_Phoenix_MotorControl_TalonFXInvertType."Clockwise", "PhoenixMotorControlDevRef"=w541) -> ("error out"=w452:errorcluster, "PhoenixMotorControlDevRef"=w453:T29)  [unwired: 7 in]
      n32 = call <vilib>:"CTRE_Phoenix_MotorControl_SetStatusFramePeriod_Enhanced.vi"("error in (no error)"=w452, "periodMs"=w435, "Status Frame"=w441, "PhoenixMotorControlDevRef"=w453) -> ("error out"=w450:errorcluster, "PhoenixMotorControlDevRef"=w451:T29)  [unwired: 6 in]
      n33 = call <vilib>:"CTRE_Phoenix_MotorControl_SetStatusFramePeriod_Enhanced.vi"("error in (no error)"=w450, "periodMs"=w435, "Status Frame"=w440, "PhoenixMotorControlDevRef"=w451) -> ("error out"=w446:errorcluster, "PhoenixMotorControlDevRef"=w447:T29)  [unwired: 6 in]
      n34 = call <vilib>:"CTRE_Phoenix_MotorControl_SetStatusFramePeriod_Enhanced.vi"("error in (no error)"=w446, "periodMs"=w435, "Status Frame"=w439, "PhoenixMotorControlDevRef"=w447) -> ("error out"=w448:errorcluster, "PhoenixMotorControlDevRef"=w449:T29)  [unwired: 6 in]
      n35 = call <vilib>:"CTRE_Phoenix_MotorControl_SetStatusFramePeriod_Enhanced.vi"("error in (no error)"=w448, "periodMs"=w435, "Status Frame"=w438, "PhoenixMotorControlDevRef"=w449) -> ("error out"=w442:errorcluster, "PhoenixMotorControlDevRef"=w443:T29)  [unwired: 6 in]
      n36 = call <vilib>:"CTRE_Phoenix_MotorControl_SetStatusFramePeriod_Enhanced.vi"("error in (no error)"=w442, "periodMs"=w435, "Status Frame"=w437, "PhoenixMotorControlDevRef"=w443) -> ("error out"=w444:errorcluster, "PhoenixMotorControlDevRef"=w445:T29)  [unwired: 6 in]
      n37 = call <vilib>:"CTRE_Phoenix_MotorControl_SetStatusFramePeriod_Enhanced.vi"("error in (no error)"=w444, "periodMs"=w435, "Status Frame"=w436, "PhoenixMotorControlDevRef"=w445) -> ("error out"=w415:errorcluster, "PhoenixMotorControlDevRef"=w414:T29)  [unwired: 6 in]
      n38 = call <vilib>:"CTRE_Phoenix_MotorControl_SetNeutralMode.vi"("error in (no error)"=w415, "Motor Control Neutral Mode"=CTRE_Phoenix_MotorControl_NeutralMode."Override to Coast", "PhoenixMotorControlDevRef"=w414) -> ("error out"=w125:errorcluster, "PhoenixMotorControlDevRef"=w126:T29)  [unwired: 7 in]
      n39 = call <vilib>:"CTRE_Phoenix_MotorControl_SetControlFramePeriod_Enhanced.vi"("error in (no error)"=w125, "periodMs"=50, "Control Frame"=w123, "MotorControl Device Ref"=w126) -> ("error out"=w124:errorcluster)  [unwired: 6 in, 1 out]
      n40 = call <vilib>:"CTRE_Phoenix_TalonFX_Open.vi"("error in"=w124, "Device Number"=u8 14) -> ("error out"=w549:errorcluster, "PhoenixMotorControlDevRef"=w550:T29)  [unwired: 8 in]
      n41 = call <vilib>:"CTRE_Phoenix_MotorControl_FactoryDefault.vi"("error in"=w549, "PhoenixMotorControlDevRef"=w550) -> ("error out"=w551:errorcluster, "PhoenixMotorControlDevRef"=w552:T29)  [unwired: 8 in]
      n42 = call <vilib>:"CTRE_Phoenix_MotorControl_RefNumRegistrySet.vi"("error in (no error)"=w551, "refnum name"="kickup", "PhoenixMotorControlDevRef"=w552) -> ("error out"=w538:errorcluster, "PhoenixMotorControlDevRef"=w539:T29)  [unwired: 7 in]
      n43 = call <vilib>:"CTRE_Phoenix_MotorControl_SetInverted_TalonFX.vi"("error in (no error)"=w538, "Invert Type"=CTRE_Phoenix_MotorControl_TalonFXInvertType."Clockwise", "PhoenixMotorControlDevRef"=w539) -> ("error out"=w536:errorcluster, "PhoenixMotorControlDevRef"=w535:T29)  [unwired: 7 in]
      n44 = call <vilib>:"CTRE_Phoenix_MotorControl_EnableVoltageCompensation.vi"("error in (no error)"=w536, "Enable Voltage Compensation?"=TRUE, "PhoenixMotorControlDevRef"=w535) -> ("error out"=w532:errorcluster, "PhoenixMotorControlDevRef"=w533:T29)  [unwired: 7 in]
      n45 = call <vilib>:"CTRE_Phoenix_MotorControl_ConfigVoltageCompensation.vi"("error in (no error)"=w532, "Saturation Voltage"=11.5, "PhoenixMotorControlDevRef"=w533) -> ("error out"=w529:errorcluster, "PhoenixMotorControlDevRef"=w530:T29)  [unwired: 7 in]
      n46 = call <vilib>:"CTRE_Phoenix_MotorControl_ConfigClosedLoopConstants.vi"("PhoenixMotorControlDevRef"=w530, "slotIdx"=0, "P"=0.06, "D"=5.0, "error in (no error)"=w529, "F"=0.0491) -> ("PhoenixMotorControlDevRef"=w417:T29, "error out"=w416:errorcluster)  [unwired: 8 in]
      n47 = call <vilib>:"CTRE_Phoenix_MotorControl_SetStatusFramePeriod_Enhanced.vi"("error in (no error)"=w416, "periodMs"=w421, "Status Frame"=w424, "PhoenixMotorControlDevRef"=w417) -> ("error out"=w433:errorcluster, "PhoenixMotorControlDevRef"=w434:T29)  [unwired: 6 in]
      n48 = call <vilib>:"CTRE_Phoenix_MotorControl_SetStatusFramePeriod_Enhanced.vi"("error in (no error)"=w433, "periodMs"=w421, "Status Frame"=w420, "PhoenixMotorControlDevRef"=w434) -> ("error out"=w429:errorcluster, "PhoenixMotorControlDevRef"=w430:T29)  [unwired: 6 in]
      n49 = call <vilib>:"CTRE_Phoenix_MotorControl_SetStatusFramePeriod_Enhanced.vi"("error in (no error)"=w429, "periodMs"=w421, "Status Frame"=w423, "PhoenixMotorControlDevRef"=w430) -> ("error out"=w431:errorcluster, "PhoenixMotorControlDevRef"=w432:T29)  [unwired: 6 in]
      n50 = call <vilib>:"CTRE_Phoenix_MotorControl_SetStatusFramePeriod_Enhanced.vi"("error in (no error)"=w431, "periodMs"=w421, "Status Frame"=w419, "PhoenixMotorControlDevRef"=w432) -> ("error out"=w425:errorcluster, "PhoenixMotorControlDevRef"=w426:T29)  [unwired: 6 in]
      n51 = call <vilib>:"CTRE_Phoenix_MotorControl_SetStatusFramePeriod_Enhanced.vi"("error in (no error)"=w425, "periodMs"=w421, "Status Frame"=w422, "PhoenixMotorControlDevRef"=w426) -> ("error out"=w427:errorcluster, "PhoenixMotorControlDevRef"=w428:T29)  [unwired: 6 in]
      n52 = call <vilib>:"CTRE_Phoenix_MotorControl_SetStatusFramePeriod_Enhanced.vi"("error in (no error)"=w427, "periodMs"=w421, "Status Frame"=w418, "PhoenixMotorControlDevRef"=w428) -> ("error out"=w308:errorcluster, "PhoenixMotorControlDevRef"=w307:T29)  [unwired: 6 in]
      n53 = call <vilib>:"CTRE_Phoenix_MotorControl_SetNeutralMode.vi"("error in (no error)"=w308, "Motor Control Neutral Mode"=CTRE_Phoenix_MotorControl_NeutralMode."Override to Coast", "PhoenixMotorControlDevRef"=w307) -> ("error out"=w305:errorcluster)  [unwired: 7 in, 1 out]
      n54 = call "Initiallize Shooters.vi"("error in"=w305) -> ("error out"=w324:errorcluster)  [unwired: 10 in]
      n55 = call <vilib>:"CTRE_Phoenix_TalonFX_Open.vi"("error in"=w324, "Device Number"=u8 43) -> ("error out"=w359:errorcluster, "PhoenixMotorControlDevRef"=w360:T29)  [unwired: 8 in]
      n56 = call <vilib>:"CTRE_Phoenix_MotorControl_FactoryDefault.vi"("error in"=w359, "PhoenixMotorControlDevRef"=w360) -> ("error out"=w361:errorcluster, "PhoenixMotorControlDevRef"=w362:T29)  [unwired: 8 in]
      n57 = call <vilib>:"CTRE_Phoenix_MotorControl_RefNumRegistrySet.vi"("error in (no error)"=w361, "refnum name"="climberWinch", "PhoenixMotorControlDevRef"=w362) -> ("error out"=w357:errorcluster, "PhoenixMotorControlDevRef"=w358:T29)  [unwired: 7 in]
      n58 = call <vilib>:"CTRE_Phoenix_MotorControl_SetInverted_TalonFX.vi"("error in (no error)"=w357, "Invert Type"=CTRE_Phoenix_MotorControl_TalonFXInvertType."Counter-Clockwise", "PhoenixMotorControlDevRef"=w358) -> ("error out"=w356:errorcluster, "PhoenixMotorControlDevRef"=w355:T29)  [unwired: 7 in]
      n59 = call <vilib>:"CTRE_Phoenix_MotorControl_EnableVoltageCompensation.vi"("error in (no error)"=w356, "Enable Voltage Compensation?"=TRUE, "PhoenixMotorControlDevRef"=w355) -> ("error out"=w352:errorcluster, "PhoenixMotorControlDevRef"=w353:T29)  [unwired: 7 in]
      n60 = call <vilib>:"CTRE_Phoenix_MotorControl_ConfigVoltageCompensation.vi"("error in (no error)"=w352, "Saturation Voltage"=11.5, "PhoenixMotorControlDevRef"=w353) -> ("error out"=w349:errorcluster, "PhoenixMotorControlDevRef"=w350:T29)  [unwired: 7 in]
      n61 = call <vilib>:"CTRE_Phoenix_MotorControl_ConfigClosedLoopConstants.vi"("PhoenixMotorControlDevRef"=w350, "slotIdx"=0, "P"=0.07, "D"=0.1, "error in (no error)"=w349, "F"=0.0) -> ("PhoenixMotorControlDevRef"=w328:T29, "error out"=w327:errorcluster)  [unwired: 8 in]
      n62 = call <vilib>:"CTRE_Phoenix_MotorControl_SetStatusFramePeriod_Enhanced.vi"("error in (no error)"=w327, "periodMs"=w332, "Status Frame"=w335, "PhoenixMotorControlDevRef"=w328) -> ("error out"=w344:errorcluster, "PhoenixMotorControlDevRef"=w345:T29)  [unwired: 6 in]
      n63 = call <vilib>:"CTRE_Phoenix_MotorControl_SetStatusFramePeriod_Enhanced.vi"("error in (no error)"=w344, "periodMs"=w332, "Status Frame"=w331, "PhoenixMotorControlDevRef"=w345) -> ("error out"=w340:errorcluster, "PhoenixMotorControlDevRef"=w341:T29)  [unwired: 6 in]
      n64 = call <vilib>:"CTRE_Phoenix_MotorControl_SetStatusFramePeriod_Enhanced.vi"("error in (no error)"=w340, "periodMs"=w332, "Status Frame"=w334, "PhoenixMotorControlDevRef"=w341) -> ("error out"=w342:errorcluster, "PhoenixMotorControlDevRef"=w343:T29)  [unwired: 6 in]
      n65 = call <vilib>:"CTRE_Phoenix_MotorControl_SetStatusFramePeriod_Enhanced.vi"("error in (no error)"=w342, "periodMs"=w332, "Status Frame"=w330, "PhoenixMotorControlDevRef"=w343) -> ("error out"=w336:errorcluster, "PhoenixMotorControlDevRef"=w337:T29)  [unwired: 6 in]
      n66 = call <vilib>:"CTRE_Phoenix_MotorControl_SetStatusFramePeriod_Enhanced.vi"("error in (no error)"=w336, "periodMs"=w332, "Status Frame"=w333, "PhoenixMotorControlDevRef"=w337) -> ("error out"=w338:errorcluster, "PhoenixMotorControlDevRef"=w339:T29)  [unwired: 6 in]
      n67 = call <vilib>:"CTRE_Phoenix_MotorControl_SetStatusFramePeriod_Enhanced.vi"("error in (no error)"=w338, "periodMs"=w332, "Status Frame"=w329, "PhoenixMotorControlDevRef"=w339) -> ("error out"=w310:errorcluster, "PhoenixMotorControlDevRef"=w311:T29)  [unwired: 6 in]
      n68 = call <vilib>:"CTRE_Phoenix_MotorControl_SetSelectedSensorPosition.vi"("error in (no error)"=w310, "New Sensor Position"=0, "PhoenixMotorControlDevRef"=w311) -> ("error out"=w120:errorcluster, "PhoenixMotorControlDevRef"=w121:T29)  [unwired: 7 in]
      n69 = call <vilib>:"CTRE_Phoenix_MotorControl_SetControlFramePeriod_Enhanced.vi"("error in (no error)"=w120, "periodMs"=50, "Control Frame"=w119, "MotorControl Device Ref"=w121) -> ("error out"=w13:errorcluster, "PhoenixMotorControlDevRef"=w12:T29)  [unwired: 6 in]
      n70 = call <vilib>:"CTRE_Phoenix_MotorControl_SetNeutralMode.vi"("error in (no error)"=w13, "Motor Control Neutral Mode"=CTRE_Phoenix_MotorControl_NeutralMode."Override to Coast", "PhoenixMotorControlDevRef"=w12) -> ("error out"=w11:errorcluster)  [unwired: 7 in, 1 out]
      n71 = call <vilib>:"CTRE_Phoenix_TalonFX_Open.vi"("error in"=w11, "Device Number"=u8 40) -> ("error out"=w50:errorcluster, "PhoenixMotorControlDevRef"=w49:T29)  [unwired: 8 in]
      n72 = call <vilib>:"CTRE_Phoenix_MotorControl_FactoryDefault.vi"("error in"=w50, "PhoenixMotorControlDevRef"=w49) -> ("error out"=w48:errorcluster, "PhoenixMotorControlDevRef"=w47:T29)  [unwired: 8 in]
      n73 = call <vilib>:"CTRE_Phoenix_MotorControl_RefNumRegistrySet.vi"("error in (no error)"=w48, "refnum name"="climberArm", "PhoenixMotorControlDevRef"=w47) -> ("error out"=w52:errorcluster, "PhoenixMotorControlDevRef"=w51:T29)  [unwired: 7 in]
      n74 = call <vilib>:"CTRE_Phoenix_MotorControl_SetInverted_TalonFX.vi"("error in (no error)"=w52, "Invert Type"=CTRE_Phoenix_MotorControl_TalonFXInvertType."Clockwise", "PhoenixMotorControlDevRef"=w51) -> ("error out"=w53:errorcluster, "PhoenixMotorControlDevRef"=w54:T29)  [unwired: 7 in]
      n75 = call <vilib>:"CTRE_Phoenix_MotorControl_EnableVoltageCompensation.vi"("error in (no error)"=w53, "Enable Voltage Compensation?"=TRUE, "PhoenixMotorControlDevRef"=w54) -> ("error out"=w57:errorcluster, "PhoenixMotorControlDevRef"=w56:T29)  [unwired: 7 in]
      n76 = call <vilib>:"CTRE_Phoenix_MotorControl_ConfigVoltageCompensation.vi"("error in (no error)"=w57, "Saturation Voltage"=11.5, "PhoenixMotorControlDevRef"=w56) -> ("error out"=w60:errorcluster, "PhoenixMotorControlDevRef"=w59:T29)  [unwired: 7 in]
      n77 = call <vilib>:"CTRE_Phoenix_MotorControl_ConfigClosedLoopConstants.vi"("PhoenixMotorControlDevRef"=w59, "slotIdx"=0, "P"=0.05, "D"=0.5, "error in (no error)"=w60, "F"=0.0) -> ("PhoenixMotorControlDevRef"=w44:T29, "error out"=w43:errorcluster)  [unwired: 8 in]
      n78 = call <vilib>:"CTRE_Phoenix_MotorControl_SetSensorPhase.vi"("error in (no error)"=w43, "PhaseSensor"=FALSE, "PhoenixMotorControlDevRef"=w44) -> ("error out"=w41:errorcluster, "PhoenixMotorControlDevRef"=w42:T29)  [unwired: 7 in]
      n79 = call <vilib>:"CTRE_Phoenix_MotorControl_SetStatusFramePeriod_Enhanced.vi"("error in (no error)"=w41, "periodMs"=w77, "Status Frame"=w74, "PhoenixMotorControlDevRef"=w42) -> ("error out"=w65:errorcluster, "PhoenixMotorControlDevRef"=w64:T29)  [unwired: 6 in]
      n80 = call <vilib>:"CTRE_Phoenix_MotorControl_SetStatusFramePeriod_Enhanced.vi"("error in (no error)"=w65, "periodMs"=w77, "Status Frame"=w78, "PhoenixMotorControlDevRef"=w64) -> ("error out"=w69:errorcluster, "PhoenixMotorControlDevRef"=w68:T29)  [unwired: 6 in]
      n81 = call <vilib>:"CTRE_Phoenix_MotorControl_SetStatusFramePeriod_Enhanced.vi"("error in (no error)"=w69, "periodMs"=w77, "Status Frame"=w75, "PhoenixMotorControlDevRef"=w68) -> ("error out"=w67:errorcluster, "PhoenixMotorControlDevRef"=w66:T29)  [unwired: 6 in]
      n82 = call <vilib>:"CTRE_Phoenix_MotorControl_SetStatusFramePeriod_Enhanced.vi"("error in (no error)"=w67, "periodMs"=w77, "Status Frame"=w79, "PhoenixMotorControlDevRef"=w66) -> ("error out"=w73:errorcluster, "PhoenixMotorControlDevRef"=w72:T29)  [unwired: 6 in]
      n83 = call <vilib>:"CTRE_Phoenix_MotorControl_SetStatusFramePeriod_Enhanced.vi"("error in (no error)"=w73, "periodMs"=w77, "Status Frame"=w76, "PhoenixMotorControlDevRef"=w72) -> ("error out"=w71:errorcluster, "PhoenixMotorControlDevRef"=w70:T29)  [unwired: 6 in]
      n84 = call <vilib>:"CTRE_Phoenix_MotorControl_SetStatusFramePeriod_Enhanced.vi"("error in (no error)"=w71, "periodMs"=w77, "Status Frame"=w80, "PhoenixMotorControlDevRef"=w70) -> ("error out"=w85:errorcluster, "PhoenixMotorControlDevRef"=w84:T29)  [unwired: 6 in]
      n85 = call <vilib>:"CTRE_Phoenix_MotorControl_SetSelectedSensorPosition.vi"("error in (no error)"=w85, "New Sensor Position"=0, "PhoenixMotorControlDevRef"=w84) -> ("error out"=w88:errorcluster, "PhoenixMotorControlDevRef"=w87:T29)  [unwired: 7 in]
      n86 = call <vilib>:"CTRE_Phoenix_MotorControl_SetControlFramePeriod_Enhanced.vi"("error in (no error)"=w88, "periodMs"=50, "Control Frame"=w89, "MotorControl Device Ref"=w87) -> ("error out"=w38:errorcluster, "PhoenixMotorControlDevRef"=w39:T29)  [unwired: 6 in]
      n87 = call <vilib>:"CTRE_Phoenix_MotorControl_ConfigPeakOutput.vi"("error in (no error)"=w38, "Reverse Peak Percent Output"=-0.28, "Forward Peak Percent Output"=0.28, "PhoenixMotorControlDevRef"=w39) -> ("error out"=w34:errorcluster, "PhoenixMotorControlDevRef"=w35:T29)  [unwired: 6 in]
      n88 = call <vilib>:"CTRE_Phoenix_MotorControl_ConfigSupplyCurrentLimit.vi"("error in (no error)"=w34, "Supply Current Limit Configuration"="Supply Current Limit Configuration", "PhoenixMotorControlDevRef"=w35) -> ("error out"=w32:errorcluster, "PhoenixMotorControlDevRef"=w31:T29)  [unwired: 7 in]
      n89 = call <vilib>:"CTRE_Phoenix_MotorControl_ConfigClosedLoopRamp.vi"("error in (no error)"=w32, "secondsFromNeutralToFull"=0.25, "PhoenixMotorControlDevRef"=w31) -> ("error out"=w28:errorcluster, "PhoenixMotorControlDevRef"=w29:T29)  [unwired: 7 in]
      n90 = call <vilib>:"CTRE_Phoenix_MotorControl_SetNeutralMode.vi"("error in (no error)"=w28, "Motor Control Neutral Mode"=CTRE_Phoenix_MotorControl_NeutralMode."Override to Coast", "PhoenixMotorControlDevRef"=w29) -> ("error out"=w26:errorcluster)  [unwired: 7 in, 1 out]
      n91 = call <vilib>:"WPI_JoystickRefNum Registry Set.vi"("error in (no error)"=w26, "refnum name"="driver", "JoystickDevRef"=w578) -> ("error out"=w93:errorcluster)  [unwired: 7 in, 1 out]
      n92 = call <vilib>:"WPI_JoystickRefNum Registry Set.vi"("error in (no error)"=w93, "refnum name"="operator", "JoystickDevRef"=w579) -> ("error out"=w92:errorcluster)  [unwired: 7 in, 1 out]
      n93 = call <vilib>:"Spark MAX Open.vi"("error in (no error)"=w92, "Device Number"=u8 11) -> ("error out"=w557:errorcluster, "MotorControlDeviceRef"=w558:T29)  [unwired: 8 in]
      n94 = call <vilib>:"Spark MAX Restore Factory Default.vi"("error in"=w557, "MotorControlDeviceRef"=w558) -> ("error out"=w556:errorcluster, "MotorControlDeviceRef"=w555:T29)  [unwired: 8 in]
      n95 = call <vilib>:"WPI_MotorControlRefNum Registry Set.vi"("error in (no error)"=w556, "refnum name"="indexer", "MotorControlDevRef"=w555) -> ("error out"=w486:errorcluster, "MotorControlDevRef"=w485:T29)  [unwired: 7 in]
      n96 = call <vilib>:"Spark MAX Set Idle Mode.vi"("error in (no error)"=w486, "Idle Mode"=Spark_MAX_Idle_Mode."Brake", "MotorControlDeviceRef in"=w485) -> ("error out"=w478:errorcluster, "MotorControlDeviceRef out"=w479:T29)  [unwired: 7 in]
      n97 = call <vilib>:"Spark MAX Set Periodic Frame Rate.vi"("error in"=w478, "Frame rate (ms)"=w474, "Frame"=Spark_MAX_Status_Frames."Status 0", "MotorControlDeviceRef"=w479) -> ("error out"=w483:errorcluster, "MotorControlDeviceRef"=w482:T29)  [unwired: 6 in]
      n98 = call <vilib>:"Spark MAX Set Periodic Frame Rate.vi"("error in"=w483, "Frame rate (ms)"=w474, "Frame"=Spark_MAX_Status_Frames."Status 1", "MotorControlDeviceRef"=w482) -> ("error out"=w481:errorcluster, "MotorControlDeviceRef"=w480:T29)  [unwired: 6 in]
      n99 = call <vilib>:"Spark MAX Set Periodic Frame Rate.vi"("error in"=w481, "Frame rate (ms)"=w474, "Frame"=Spark_MAX_Status_Frames."Status 2", "MotorControlDeviceRef"=w480) -> ("error out"=w411:errorcluster, "MotorControlDeviceRef"=w412:T29)  [unwired: 6 in]
      n100 = call <vilib>:"Spark MAX Set Motor Type.vi"("error in (no error)"=w411, "Motor Type"=Spark_MAX_Motor_Type."Brushless", "MotorControlDevRef"=w412) -> ("error out"=w409:errorcluster, "MotorControlDeviceRef"=w410:T29)  [unwired: 7 in]
      n101 = call <vilib>:"Spark MAX Burn Flash.vi"("error in"=w409, "MotorControlDeviceRef"=w410) -> ("error out"=w322:errorcluster)  [unwired: 8 in, 1 out]
      n102 = call <vilib>:"Spark MAX Open.vi"("error in (no error)"=w322, "Invert"=FALSE, "Device Number"=u8 10) -> ("error out"=w503:errorcluster, "MotorControlDeviceRef"=w504:T29)  [unwired: 7 in]
      n103 = call <vilib>:"WPI_MotorControlRefNum Registry Set.vi"("error in (no error)"=w503, "refnum name"="turretAngle", "MotorControlDevRef"=w504) -> ("error out"=w524:errorcluster, "MotorControlDevRef"=w523:T29)  [unwired: 7 in]
      n104 = call <vilib>:"Spark MAX Set Sensor Position.vi"("Sensor Type (Hall Sensor)"=Spark_MAX_Sensor_Type."Hall Sensor", "error in"=w524, "Position"=0.0, "MotorControlDeviceRef"=w523) -> ("error out"=w518:errorcluster, "MotorControlDeviceRef"=w517:T29)  [unwired: 6 in]
      n105 = call <vilib>:"Spark MAX Set Conversion Factors.vi"("error in (no error)"=w518, "Position Factor (1)"=42.0, "MotorControlDeviceRef in"=w517) -> ("error out"=w514:errorcluster, "MotorControlDeviceRef out"=w513:T29)  [unwired: 7 in]
      n106 = call <vilib>:"Spark MAX Set Voltage Compensation.vi"("error in (no error)"=w514, "Nominal Voltage"=11.5, "MotorControlDeviceRef in"=w513) -> ("error out"=w501:errorcluster, "MotorControlDeviceRef out"=w502:T29)  [unwired: 7 in]
      n107 = call <vilib>:"Spark MAX Set Output Advanced.vi"("error in (no error)"=w501, "Control Mode"=Spark_MAX_Control_Type."Position", "Setpoint"=0.0, "MotorControlDevRef"=w502) -> ("error out"=w493:errorcluster, "MotorControlDevRef"=w494:T29)  [unwired: 6 in]
      n108 = call <vilib>:"Spark MAX Set PIDF Constants.vi"("error in"=w493, "PIDF Slot"=0, "PID Constants"=T9 {"P Gain"=0.01, "I Gain"=0.0, "D Gain"=0.0, "F Gain"=0.0, "I Zone"=0.0, "Min Output"=-0.7, "Max Output"=0.7}, "MotorControlDeviceRef"=w494) -> ("error out"=w454:errorcluster, "MotorControlDeviceRef"=w455:T29)  [unwired: 6 in]
      n109 = call <vilib>:"Spark MAX Set Periodic Frame Rate.vi"("error in"=w454, "Frame rate (ms)"=w458, "Frame"=Spark_MAX_Status_Frames."Status 0", "MotorControlDeviceRef"=w455) -> ("error out"=w465:errorcluster, "MotorControlDeviceRef"=w464:T29)  [unwired: 6 in]
      n110 = call <vilib>:"Spark MAX Set Periodic Frame Rate.vi"("error in"=w465, "Frame rate (ms)"=w458, "Frame"=Spark_MAX_Status_Frames."Status 1", "MotorControlDeviceRef"=w464) -> ("error out"=w463:errorcluster, "MotorControlDeviceRef"=w462:T29)  [unwired: 6 in]
      n111 = call <vilib>:"Spark MAX Set Periodic Frame Rate.vi"("error in"=w463, "Frame rate (ms)"=w458, "Frame"=Spark_MAX_Status_Frames."Status 2", "MotorControlDeviceRef"=w462) -> ("error out"=w405:errorcluster, "MotorControlDeviceRef"=w407:T29)  [unwired: 6 in]
      n112 = call <vilib>:"Spark MAX Set Motor Type.vi"("error in (no error)"=w405, "Motor Type"=Spark_MAX_Motor_Type."Brushless", "MotorControlDevRef"=w407) -> ("error out"=w404:errorcluster, "MotorControlDeviceRef"=w406:T29)  [unwired: 7 in]
      n113 = call <vilib>:"Spark MAX Burn Flash.vi"("error in"=w404, "MotorControlDeviceRef"=w406) -> ("error out"=w321:errorcluster)  [unwired: 8 in, 1 out]
      n114 = call <vilib>:"Spark MAX Open.vi"("error in (no error)"=w321, "Invert"=TRUE, "Device Number"=u8 1) -> ("error out"=w505:errorcluster, "MotorControlDeviceRef"=w506:T29)  [unwired: 7 in]
      n115 = call <vilib>:"WPI_MotorControlRefNum Registry Set.vi"("error in (no error)"=w505, "refnum name"="hoodAngle", "MotorControlDevRef"=w506) -> ("error out"=w24:errorcluster, "MotorControlDevRef"=w25:T29)  [unwired: 7 in]
      n116 = call <vilib>:"Spark MAX Set Conversion Factors.vi"("error in (no error)"=w24, "Position Factor (1)"=42.0, "MotorControlDeviceRef in"=w25) -> ("error out"=w512:errorcluster, "MotorControlDeviceRef out"=w511:T29)  [unwired: 7 in]
      n117 = call <vilib>:"Spark MAX Set Voltage Compensation.vi"("error in (no error)"=w512, "Nominal Voltage"=11.5, "MotorControlDeviceRef in"=w511) -> ("error out"=w498:errorcluster, "MotorControlDeviceRef out"=w499:T29)  [unwired: 7 in]
      n118 = call <vilib>:"Spark MAX Set Output Advanced.vi"("error in (no error)"=w498, "Control Mode"=Spark_MAX_Control_Type."Position", "Setpoint"=0.0, "MotorControlDevRef"=w499) -> ("error out"=w492:errorcluster, "MotorControlDevRef"=w491:T29)  [unwired: 6 in]
      n119 = call <vilib>:"Spark MAX Set PIDF Constants.vi"("error in"=w492, "PIDF Slot"=0, "PID Constants"=T9 {"P Gain"=0.009, "I Gain"=0.0, "D Gain"=0.0, "F Gain"=0.0, "I Zone"=0.0, "Min Output"=-0.6, "Max Output"=0.6}, "MotorControlDeviceRef"=w491) -> ("error out"=w456:errorcluster, "MotorControlDeviceRef"=w457:T29)  [unwired: 6 in]
      n120 = call <vilib>:"Spark MAX Set Periodic Frame Rate.vi"("error in"=w456, "Frame rate (ms)"=w466, "Frame"=Spark_MAX_Status_Frames."Status 0", "MotorControlDeviceRef"=w457) -> ("error out"=w473:errorcluster, "MotorControlDeviceRef"=w472:T29)  [unwired: 6 in]
      n121 = call <vilib>:"Spark MAX Set Periodic Frame Rate.vi"("error in"=w473, "Frame rate (ms)"=w466, "Frame"=Spark_MAX_Status_Frames."Status 1", "MotorControlDeviceRef"=w472) -> ("error out"=w471:errorcluster, "MotorControlDeviceRef"=w470:T29)  [unwired: 6 in]
      n122 = call <vilib>:"Spark MAX Set Periodic Frame Rate.vi"("error in"=w471, "Frame rate (ms)"=w466, "Frame"=Spark_MAX_Status_Frames."Status 2", "MotorControlDeviceRef"=w470) -> ("error out"=w400:errorcluster, "MotorControlDeviceRef"=w402:T29)  [unwired: 6 in]
      n123 = call <vilib>:"Spark MAX Set Motor Type.vi"("error in (no error)"=w400, "Motor Type"=Spark_MAX_Motor_Type."Brushless", "MotorControlDevRef"=w402) -> ("error out"=w399:errorcluster, "MotorControlDeviceRef"=w401:T29)  [unwired: 7 in]
      n124 = call <vilib>:"Spark MAX Burn Flash.vi"("error in"=w399, "MotorControlDeviceRef"=w401) -> ("error out"=w22:errorcluster, "MotorControlDeviceRef"=w23:T29)  [unwired: 8 in]
      n125 = call <vilib>:"Spark MAX Set Sensor Position.vi"("Sensor Type (Hall Sensor)"=Spark_MAX_Sensor_Type."Hall Sensor", "error in"=w22, "Position"=0.0, "MotorControlDeviceRef"=w23) -> ("error out"=w21:errorcluster)  [unwired: 6 in, 1 out]
      n126 = call <vilib>:"Spark MAX Open.vi"("error in (no error)"=w21, "Invert"=FALSE, "Device Number"=u8 41) -> ("error out"=w385:errorcluster, "MotorControlDeviceRef"=w386:T29)  [unwired: 7 in]
      n127 = call <vilib>:"WPI_MotorControlRefNum Registry Set.vi"("error in (no error)"=w385, "refnum name"="intakeLift", "MotorControlDevRef"=w386) -> ("error out"=w14:errorcluster, "MotorControlDevRef"=w15:T29)  [unwired: 7 in]
      n128 = call <vilib>:"Spark MAX Set Conversion Factors.vi"("error in (no error)"=w14, "Position Factor (1)"=42.0, "MotorControlDeviceRef in"=w15) -> ("error out"=w390:errorcluster, "MotorControlDeviceRef out"=w389:T29)  [unwired: 7 in]
      n129 = call <vilib>:"Spark MAX Set Voltage Compensation.vi"("error in (no error)"=w390, "Nominal Voltage"=11.5, "MotorControlDeviceRef in"=w389) -> ("error out"=w383:errorcluster, "MotorControlDeviceRef out"=w384:T29)  [unwired: 7 in]
      n130 = call <vilib>:"Spark MAX Set Output Advanced.vi"("error in (no error)"=w383, "Control Mode"=Spark_MAX_Control_Type."Position", "Setpoint"=0.0, "MotorControlDevRef"=w384) -> ("error out"=w381:errorcluster, "MotorControlDevRef"=w380:T29)  [unwired: 6 in]
      n131 = call <vilib>:"Spark MAX Set PIDF Constants.vi"("error in"=w381, "PIDF Slot"=0, "PID Constants"=T9 {"P Gain"=0.003, "I Gain"=0.0, "D Gain"=0.5, "F Gain"=0.0, "I Zone"=0.0, "Min Output"=-0.7, "Max Output"=0.7}, "MotorControlDeviceRef"=w380) -> ("error out"=w368:errorcluster, "MotorControlDeviceRef"=w369:T29)  [unwired: 6 in]
      n132 = call <vilib>:"Spark MAX Set Periodic Frame Rate.vi"("error in"=w368, "Frame rate (ms)"=w370, "Frame"=Spark_MAX_Status_Frames."Status 0", "MotorControlDeviceRef"=w369) -> ("error out"=w377:errorcluster, "MotorControlDeviceRef"=w376:T29)  [unwired: 6 in]
      n133 = call <vilib>:"Spark MAX Set Periodic Frame Rate.vi"("error in"=w377, "Frame rate (ms)"=w370, "Frame"=Spark_MAX_Status_Frames."Status 1", "MotorControlDeviceRef"=w376) -> ("error out"=w375:errorcluster, "MotorControlDeviceRef"=w374:T29)  [unwired: 6 in]
      n134 = call <vilib>:"Spark MAX Set Periodic Frame Rate.vi"("error in"=w375, "Frame rate (ms)"=w370, "Frame"=Spark_MAX_Status_Frames."Status 2", "MotorControlDeviceRef"=w374) -> ("error out"=w366:errorcluster, "MotorControlDeviceRef"=w367:T29)  [unwired: 6 in]
      n135 = call <vilib>:"Spark MAX Set Motor Type.vi"("error in (no error)"=w366, "Motor Type"=Spark_MAX_Motor_Type."Brushless", "MotorControlDevRef"=w367) -> ("error out"=w319:errorcluster, "MotorControlDeviceRef"=w320:T29)  [unwired: 7 in]
      n136 = call <vilib>:"Spark MAX Set Current Limit.vi"("error in (no error)"=w319, "Current Limit A (100)"=sgl 5.0, "MotorControlDeviceRef in"=w320) -> ("error out"=w315:errorcluster, "MotorControlDeviceRef out"=w317:T29)  [unwired: 7 in]
      n137 = call <vilib>:"Spark MAX Set Closed Loop Ramp Rate.vi"("error in (no error)"=w315, "Seconds from neutral to full (0)"=sgl 0.75, "MotorControlDeviceRef in"=w317) -> ("error out"=w314:errorcluster, "MotorControlDeviceRef"=w316:T29)  [unwired: 7 in]
      n138 = call <vilib>:"Spark MAX Burn Flash.vi"("error in"=w314, "MotorControlDeviceRef"=w316) -> ("error out"=w17:errorcluster, "MotorControlDeviceRef"=w18:T29)  [unwired: 8 in]
      n139 = call <vilib>:"Spark MAX Set Sensor Position.vi"("Sensor Type (Hall Sensor)"=Spark_MAX_Sensor_Type."Hall Sensor", "error in"=w17, "Position"=0.0, "MotorControlDeviceRef"=w18) -> ("error out"=w16:errorcluster)  [unwired: 6 in, 1 out]
      n140 = call <vilib>:"Spark MAX Open.vi"("error in (no error)"=w16, "Invert"=FALSE, "Device Number"=u8 4) -> ("error out"=w304:errorcluster, "MotorControlDeviceRef"=w303:T29)  [unwired: 7 in]
      n141 = call <vilib>:"WPI_MotorControlRefNum Registry Set.vi"("error in (no error)"=w304, "refnum name"="leftFrontAngle", "MotorControlDevRef"=w303) -> ("error out"=w277:errorcluster, "MotorControlDevRef"=w278:T29)  [unwired: 7 in]
      n142 = call <vilib>:"Spark MAX Set Smart Current Limit.vi"("Linearized Limit Enabled (F)"=TRUE, "error in (no error)"=w277, "Primay Current Limit (80A)"=40.0, "MotorControlDeviceRef in"=w278) -> ("error out"=w302:errorcluster, "MotorControlDeviceRef out"=w301:T29)  [unwired: 6 in]
      n143 = call <vilib>:"Spark MAX Set Feedback Sensor Type.vi"("error in (no error)"=w302, "Sensor Type"=Spark_MAX_Sensor_Type."Hall Sensor", "MotorControlDevRef"=w301) -> ("error out"=w300:errorcluster, "MotorControlDeviceRef"=w299:T29)  [unwired: 7 in]
      n144 = call <vilib>:"Spark MAX Set Motor Type.vi"("error in (no error)"=w300, "Motor Type"=Spark_MAX_Motor_Type."Brushless", "MotorControlDevRef"=w299) -> ("error out"=w298:errorcluster, "MotorControlDeviceRef"=w297:T29)  [unwired: 7 in]
      n145 = call <vilib>:"Spark MAX Set Conversion Factors.vi"("error in (no error)"=w298, "MotorControlDeviceRef in"=w297) -> ("error out"=w296:errorcluster, "MotorControlDeviceRef out"=w295:T29)  [unwired: 8 in]
      n146 = call <vilib>:"Spark MAX Set Sensor Position.vi"("error in"=w296, "Position"=0.0, "MotorControlDeviceRef"=w295) -> ("error out"=w294:errorcluster, "MotorControlDeviceRef"=w293:T29)  [unwired: 7 in]
      n147 = call <vilib>:"Spark MAX Set Closed Loop Ramp Rate.vi"("error in (no error)"=w294, "Seconds from neutral to full (0)"=sgl 0.0, "MotorControlDeviceRef in"=w293) -> ("error out"=w292:errorcluster, "MotorControlDeviceRef"=w291:T29)  [unwired: 7 in]
      n148 = call <vilib>:"Spark MAX Set Voltage Compensation.vi"("error in (no error)"=w292, "Nominal Voltage"=11.5, "MotorControlDeviceRef in"=w291) -> ("error out"=w290:errorcluster, "MotorControlDeviceRef out"=w289:T29)  [unwired: 7 in]
      n149 = call <vilib>:"Spark MAX Set Idle Mode.vi"("error in (no error)"=w290, "Idle Mode"=Spark_MAX_Idle_Mode."Brake", "MotorControlDeviceRef in"=w289) -> ("error out"=w281:errorcluster, "MotorControlDeviceRef out"=w282:T29)  [unwired: 7 in]
      n150 = call <vilib>:"Spark MAX Set Periodic Frame Rate.vi"("error in"=w281, "Frame rate (ms)"=w134, "Frame"=Spark_MAX_Status_Frames."Status 0", "MotorControlDeviceRef"=w282) -> ("error out"=w288:errorcluster, "MotorControlDeviceRef"=w287:T29)  [unwired: 6 in]
      n151 = call <vilib>:"Spark MAX Set Periodic Frame Rate.vi"("error in"=w288, "Frame rate (ms)"=w134, "Frame"=Spark_MAX_Status_Frames."Status 1", "MotorControlDeviceRef"=w287) -> ("error out"=w286:errorcluster, "MotorControlDeviceRef"=w285:T29)  [unwired: 6 in]
      n152 = call <vilib>:"Spark MAX Set Periodic Frame Rate.vi"("error in"=w286, "Frame rate (ms)"=w134, "Frame"=Spark_MAX_Status_Frames."Status 2", "MotorControlDeviceRef"=w285) -> ("error out"=w269:errorcluster, "MotorControlDeviceRef"=w270:T29)  [unwired: 6 in]
      n153 = call <vilib>:"Spark MAX Set Periodic Frame Rate.vi"("error in"=w269, "Frame rate (ms)"=w134, "Frame"=Spark_MAX_Status_Frames."Status 3", "MotorControlDeviceRef"=w270) -> ("error out"=w266:errorcluster, "MotorControlDeviceRef"=w267:T29)  [unwired: 6 in]
      n154 = call <vilib>:"Spark MAX Burn Flash.vi"("error in"=w266, "MotorControlDeviceRef"=w267) -> ("error out"=w137:errorcluster)  [unwired: 8 in, 1 out]
      n155 = call <vilib>:"Spark MAX Open.vi"("error in (no error)"=w137, "Invert"=FALSE, "Device Number"=u8 5) -> ("error out"=w224:errorcluster, "MotorControlDeviceRef"=w225:T29)  [unwired: 7 in]
      n156 = call <vilib>:"WPI_MotorControlRefNum Registry Set.vi"("error in (no error)"=w224, "refnum name"="rightFrontAngle", "MotorControlDevRef"=w225) -> ("error out"=w252:errorcluster, "MotorControlDevRef"=w251:T29)  [unwired: 7 in]
      n157 = call <vilib>:"Spark MAX Set Smart Current Limit.vi"("Linearized Limit Enabled (F)"=TRUE, "error in (no error)"=w252, "Primay Current Limit (80A)"=40.0, "MotorControlDeviceRef in"=w251) -> ("error out"=w226:errorcluster, "MotorControlDeviceRef out"=w227:T29)  [unwired: 6 in]
      n158 = call <vilib>:"Spark MAX Set Feedback Sensor Type.vi"("error in (no error)"=w226, "Sensor Type"=Spark_MAX_Sensor_Type."Hall Sensor", "MotorControlDevRef"=w227) -> ("error out"=w228:errorcluster, "MotorControlDeviceRef"=w229:T29)  [unwired: 7 in]
      n159 = call <vilib>:"Spark MAX Set Motor Type.vi"("error in (no error)"=w228, "Motor Type"=Spark_MAX_Motor_Type."Brushless", "MotorControlDevRef"=w229) -> ("error out"=w230:errorcluster, "MotorControlDeviceRef"=w231:T29)  [unwired: 7 in]
      n160 = call <vilib>:"Spark MAX Set Conversion Factors.vi"("error in (no error)"=w230, "MotorControlDeviceRef in"=w231) -> ("error out"=w232:errorcluster, "MotorControlDeviceRef out"=w233:T29)  [unwired: 8 in]
      n161 = call <vilib>:"Spark MAX Set Sensor Position.vi"("error in"=w232, "Position"=0.0, "MotorControlDeviceRef"=w233) -> ("error out"=w234:errorcluster, "MotorControlDeviceRef"=w235:T29)  [unwired: 7 in]
      n162 = call <vilib>:"Spark MAX Set Closed Loop Ramp Rate.vi"("error in (no error)"=w234, "Seconds from neutral to full (0)"=sgl 0.0, "MotorControlDeviceRef in"=w235) -> ("error out"=w236:errorcluster, "MotorControlDeviceRef"=w237:T29)  [unwired: 7 in]
      n163 = call <vilib>:"Spark MAX Set Voltage Compensation.vi"("error in (no error)"=w236, "Nominal Voltage"=11.5, "MotorControlDeviceRef in"=w237) -> ("error out"=w238:errorcluster, "MotorControlDeviceRef out"=w239:T29)  [unwired: 7 in]
      n164 = call <vilib>:"Spark MAX Set Idle Mode.vi"("error in (no error)"=w238, "Idle Mode"=Spark_MAX_Idle_Mode."Brake", "MotorControlDeviceRef in"=w239) -> ("error out"=w248:errorcluster, "MotorControlDeviceRef out"=w247:T29)  [unwired: 7 in]
      n165 = call <vilib>:"Spark MAX Set Periodic Frame Rate.vi"("error in"=w248, "Frame rate (ms)"=w133, "Frame"=Spark_MAX_Status_Frames."Status 0", "MotorControlDeviceRef"=w247) -> ("error out"=w241:errorcluster, "MotorControlDeviceRef"=w242:T29)  [unwired: 6 in]
      n166 = call <vilib>:"Spark MAX Set Periodic Frame Rate.vi"("error in"=w241, "Frame rate (ms)"=w133, "Frame"=Spark_MAX_Status_Frames."Status 1", "MotorControlDeviceRef"=w242) -> ("error out"=w243:errorcluster, "MotorControlDeviceRef"=w244:T29)  [unwired: 6 in]
      n167 = call <vilib>:"Spark MAX Set Periodic Frame Rate.vi"("error in"=w243, "Frame rate (ms)"=w133, "Frame"=Spark_MAX_Status_Frames."Status 2", "MotorControlDeviceRef"=w244) -> ("error out"=w260:errorcluster, "MotorControlDeviceRef"=w259:T29)  [unwired: 6 in]
      n168 = call <vilib>:"Spark MAX Set Periodic Frame Rate.vi"("error in"=w260, "Frame rate (ms)"=w133, "Frame"=Spark_MAX_Status_Frames."Status 3", "MotorControlDeviceRef"=w259) -> ("error out"=w263:errorcluster, "MotorControlDeviceRef"=w262:T29)  [unwired: 6 in]
      n169 = call <vilib>:"Spark MAX Burn Flash.vi"("error in"=w263, "MotorControlDeviceRef"=w262) -> ("error out"=w136:errorcluster)  [unwired: 8 in, 1 out]
      n170 = call <vilib>:"Spark MAX Open.vi"("error in (no error)"=w136, "Invert"=FALSE, "Device Number"=u8 3) -> ("error out"=w183:errorcluster, "MotorControlDeviceRef"=w184:T29)  [unwired: 7 in]
      n171 = call <vilib>:"WPI_MotorControlRefNum Registry Set.vi"("error in (no error)"=w183, "refnum name"="leftRearAngle", "MotorControlDevRef"=w184) -> ("error out"=w211:errorcluster, "MotorControlDevRef"=w210:T29)  [unwired: 7 in]
      n172 = call <vilib>:"Spark MAX Set Smart Current Limit.vi"("Linearized Limit Enabled (F)"=TRUE, "error in (no error)"=w211, "Primay Current Limit (80A)"=40.0, "MotorControlDeviceRef in"=w210) -> ("error out"=w185:errorcluster, "MotorControlDeviceRef out"=w186:T29)  [unwired: 6 in]
      n173 = call <vilib>:"Spark MAX Set Feedback Sensor Type.vi"("error in (no error)"=w185, "Sensor Type"=Spark_MAX_Sensor_Type."Hall Sensor", "MotorControlDevRef"=w186) -> ("error out"=w187:errorcluster, "MotorControlDeviceRef"=w188:T29)  [unwired: 7 in]
      n174 = call <vilib>:"Spark MAX Set Motor Type.vi"("error in (no error)"=w187, "Motor Type"=Spark_MAX_Motor_Type."Brushless", "MotorControlDevRef"=w188) -> ("error out"=w189:errorcluster, "MotorControlDeviceRef"=w190:T29)  [unwired: 7 in]
      n175 = call <vilib>:"Spark MAX Set Conversion Factors.vi"("error in (no error)"=w189, "MotorControlDeviceRef in"=w190) -> ("error out"=w191:errorcluster, "MotorControlDeviceRef out"=w192:T29)  [unwired: 8 in]
      n176 = call <vilib>:"Spark MAX Set Sensor Position.vi"("error in"=w191, "Position"=0.0, "MotorControlDeviceRef"=w192) -> ("error out"=w193:errorcluster, "MotorControlDeviceRef"=w194:T29)  [unwired: 7 in]
      n177 = call <vilib>:"Spark MAX Set Closed Loop Ramp Rate.vi"("error in (no error)"=w193, "Seconds from neutral to full (0)"=sgl 0.0, "MotorControlDeviceRef in"=w194) -> ("error out"=w195:errorcluster, "MotorControlDeviceRef"=w196:T29)  [unwired: 7 in]
      n178 = call <vilib>:"Spark MAX Set Voltage Compensation.vi"("error in (no error)"=w195, "Nominal Voltage"=11.5, "MotorControlDeviceRef in"=w196) -> ("error out"=w197:errorcluster, "MotorControlDeviceRef out"=w198:T29)  [unwired: 7 in]
      n179 = call <vilib>:"Spark MAX Set Idle Mode.vi"("error in (no error)"=w197, "Idle Mode"=Spark_MAX_Idle_Mode."Brake", "MotorControlDeviceRef in"=w198) -> ("error out"=w207:errorcluster, "MotorControlDeviceRef out"=w206:T29)  [unwired: 7 in]
      n180 = call <vilib>:"Spark MAX Set Periodic Frame Rate.vi"("error in"=w207, "Frame rate (ms)"=w132, "Frame"=Spark_MAX_Status_Frames."Status 0", "MotorControlDeviceRef"=w206) -> ("error out"=w200:errorcluster, "MotorControlDeviceRef"=w201:T29)  [unwired: 6 in]
      n181 = call <vilib>:"Spark MAX Set Periodic Frame Rate.vi"("error in"=w200, "Frame rate (ms)"=w132, "Frame"=Spark_MAX_Status_Frames."Status 1", "MotorControlDeviceRef"=w201) -> ("error out"=w202:errorcluster, "MotorControlDeviceRef"=w203:T29)  [unwired: 6 in]
      n182 = call <vilib>:"Spark MAX Set Periodic Frame Rate.vi"("error in"=w202, "Frame rate (ms)"=w132, "Frame"=Spark_MAX_Status_Frames."Status 2", "MotorControlDeviceRef"=w203) -> ("error out"=w219:errorcluster, "MotorControlDeviceRef"=w218:T29)  [unwired: 6 in]
      n183 = call <vilib>:"Spark MAX Set Periodic Frame Rate.vi"("error in"=w219, "Frame rate (ms)"=w132, "Frame"=Spark_MAX_Status_Frames."Status 3", "MotorControlDeviceRef"=w218) -> ("error out"=w222:errorcluster, "MotorControlDeviceRef"=w221:T29)  [unwired: 6 in]
      n184 = call <vilib>:"Spark MAX Burn Flash.vi"("error in"=w222, "MotorControlDeviceRef"=w221) -> ("error out"=w135:errorcluster)  [unwired: 8 in, 1 out]
      n185 = call <vilib>:"Spark MAX Open.vi"("error in (no error)"=w135, "Invert"=FALSE, "Device Number"=u8 9) -> ("error out"=w142:errorcluster, "MotorControlDeviceRef"=w143:T29)  [unwired: 7 in]
      n186 = call <vilib>:"WPI_MotorControlRefNum Registry Set.vi"("error in (no error)"=w142, "refnum name"="rightRearAngle", "MotorControlDevRef"=w143) -> ("error out"=w170:errorcluster, "MotorControlDevRef"=w169:T29)  [unwired: 7 in]
      n187 = call <vilib>:"Spark MAX Set Smart Current Limit.vi"("Linearized Limit Enabled (F)"=TRUE, "error in (no error)"=w170, "Primay Current Limit (80A)"=40.0, "MotorControlDeviceRef in"=w169) -> ("error out"=w144:errorcluster, "MotorControlDeviceRef out"=w145:T29)  [unwired: 6 in]
      n188 = call <vilib>:"Spark MAX Set Feedback Sensor Type.vi"("error in (no error)"=w144, "Sensor Type"=Spark_MAX_Sensor_Type."Hall Sensor", "MotorControlDevRef"=w145) -> ("error out"=w146:errorcluster, "MotorControlDeviceRef"=w147:T29)  [unwired: 7 in]
      n189 = call <vilib>:"Spark MAX Set Motor Type.vi"("error in (no error)"=w146, "Motor Type"=Spark_MAX_Motor_Type."Brushless", "MotorControlDevRef"=w147) -> ("error out"=w148:errorcluster, "MotorControlDeviceRef"=w149:T29)  [unwired: 7 in]
      n190 = call <vilib>:"Spark MAX Set Conversion Factors.vi"("error in (no error)"=w148, "MotorControlDeviceRef in"=w149) -> ("error out"=w150:errorcluster, "MotorControlDeviceRef out"=w151:T29)  [unwired: 8 in]
      n191 = call <vilib>:"Spark MAX Set Sensor Position.vi"("error in"=w150, "Position"=0.0, "MotorControlDeviceRef"=w151) -> ("error out"=w152:errorcluster, "MotorControlDeviceRef"=w153:T29)  [unwired: 7 in]
      n192 = call <vilib>:"Spark MAX Set Closed Loop Ramp Rate.vi"("error in (no error)"=w152, "Seconds from neutral to full (0)"=sgl 0.0, "MotorControlDeviceRef in"=w153) -> ("error out"=w154:errorcluster, "MotorControlDeviceRef"=w155:T29)  [unwired: 7 in]
      n193 = call <vilib>:"Spark MAX Set Voltage Compensation.vi"("error in (no error)"=w154, "Nominal Voltage"=11.5, "MotorControlDeviceRef in"=w155) -> ("error out"=w156:errorcluster, "MotorControlDeviceRef out"=w157:T29)  [unwired: 7 in]
      n194 = call <vilib>:"Spark MAX Set Idle Mode.vi"("error in (no error)"=w156, "Idle Mode"=Spark_MAX_Idle_Mode."Brake", "MotorControlDeviceRef in"=w157) -> ("error out"=w166:errorcluster, "MotorControlDeviceRef out"=w165:T29)  [unwired: 7 in]
      n195 = call <vilib>:"Spark MAX Set Periodic Frame Rate.vi"("error in"=w166, "Frame rate (ms)"=w131, "Frame"=Spark_MAX_Status_Frames."Status 0", "MotorControlDeviceRef"=w165) -> ("error out"=w159:errorcluster, "MotorControlDeviceRef"=w160:T29)  [unwired: 6 in]
      n196 = call <vilib>:"Spark MAX Set Periodic Frame Rate.vi"("error in"=w159, "Frame rate (ms)"=w131, "Frame"=Spark_MAX_Status_Frames."Status 1", "MotorControlDeviceRef"=w160) -> ("error out"=w161:errorcluster, "MotorControlDeviceRef"=w162:T29)  [unwired: 6 in]
      n197 = call <vilib>:"Spark MAX Set Periodic Frame Rate.vi"("error in"=w161, "Frame rate (ms)"=w131, "Frame"=Spark_MAX_Status_Frames."Status 2", "MotorControlDeviceRef"=w162) -> ("error out"=w178:errorcluster, "MotorControlDeviceRef"=w177:T29)  [unwired: 6 in]
      n198 = call <vilib>:"Spark MAX Set Periodic Frame Rate.vi"("error in"=w178, "Frame rate (ms)"=w131, "Frame"=Spark_MAX_Status_Frames."Status 3", "MotorControlDeviceRef"=w177) -> ("error out"=w181:errorcluster, "MotorControlDeviceRef"=w180:T29)  [unwired: 6 in]
      n199 = call <vilib>:"Spark MAX Burn Flash.vi"("error in"=w181, "MotorControlDeviceRef"=w180) -> ("error out"=w91:errorcluster)  [unwired: 8 in, 1 out]
    }
  }
  n200 = global write "Robot Global Data.vi" "Robot Mode"(WPI_DriverStationRobotMode2."Autonomous Disabled" ("Robot Mode")) -> ()
  "error out" <- w1
